vi "main_grid_forming_PQ.vi"() -> ()   [LabVIEW 2021]
uses:
  <vilib>/xnet/xnet.llb/XNET Frame CAN.ctl
  <vilib>/xnet/xnet.llb/XNET Frame Type CAN.ctl
  Helper functions/General Purpose/references.ctl
  Helper functions/General Purpose/measurements.ctl
  Helper functions/Time-sync/time_sync/TypeDef/Synch_shift--cluster.ctl
  <vilib>/Platform/TimedLoop/XDataNode/timing_clust.ctl
  <vilib>/Platform/TimedLoop/XDataNode/nitl_modes.ctl
  <vilib>/Platform/TimedLoop/XDataNode/wakeup.ctl
  Helper functions/communication/AFE_froming_Central.ctl
  Helper functions/communication/AFE_froming_Central_Info.ctl
  Helper functions/communication/AFE_froming_Central_Data.ctl
  <vilib>/xnet/xnet.llb/XNET Write (Frame CAN).vi
  <vilib>/xnet/xnet.llb/XNET Read (Frame CAN).vi
  <vilib>/Platform/TimedLoop/XDataNode/XDataNode.xnode
  <vilib>/Platform/TimedLoop/XDataNode/XDNodeRunTimeDep.lvlib
  <userlib>/_OpenG.lib/boolean/boolean.llb/openg_boolean__ogtk.lvlib
panel:
  in  "P2 bias":dbl
  in  "Calibration 2":T1={"IC1_Q_gain"=0.99511, "IC1_Q_bias"=-110.0, "IC2_Q_gain"=1.289, "IC2_Q_bias"=-368.5, "IC3_Q_gain"=1.003, "IC3_Q_bias"=-176.0, "IC2_P_gain"=1.2368, "IC2_P_bias"=1804.5, "IC3_P_gain"=0.9849, "IC3_P_bias"=1434.5}
  in  "Calibration":T1={"IC1_Q_gain"=0.997, "IC1_Q_bias"=-125.0, "IC2_Q_gain"=1.2829, "IC2_Q_bias"=-381.0, "IC3_Q_gain"=1.02, "IC3_Q_bias"=-252.4, "IC2_P_gain"=1.2775, "IC2_P_bias"=1561.0, "IC3_P_gain"=0.9939, "IC3_P_bias"=1271.0}
  in  "Q2 bias":dbl
  in  "delta V":dbl format="%#_13g"
  in  "delta f":dbl=0.005800000000000027 format="%#_13g"
  in  "biasQ4":dbl=200.0
  in  "biasV4":dbl
  in  "biasV1":dbl=0.6
  out "time_afe":timestamp
  out "start following 1 pre":bool
  out "Synch Monitor":string[][](table)
  in  "Loop Time":u32=125
  out "Error out":errorcluster
  in  "Timeout [ms]":i32=3000
  out "Offset from TR (ns)":dbl
  out "Status Out":T2
  out "CAN OUT":T3[](array[typedef]) {"payload" format="%x"; "timestamp" format="%<%.7X\n%x>T"; "type" items=["CAN Data"=0, "CAN Remote"=1, "CAN Bus Error"=2, "CAN 2.0 Data"=8, "CAN FD Data"=16, "CAN FD+BRS Data"=24, "J1939 Data"=192, "Delay"=224, "Log Trigger"=225, "Start Trigger"=226]; "identifier" format="%x"}
  in  "freq 1":dbl=50.0
  in  "Vabs 1":dbl=230.0
  in  "Varg 1":dbl
  in  "Start following 1":bool
  out "Forming 2":bool
  out "Forming 1":bool
  in  "Start forming 1":bool
  out "current time":timestamp
  in  "measurements":T5
  in  "references":T6
  in  "To ACT CH 4":bool
  in  "To ACT CH 3":bool
  in  "To ACT CH 2":bool
  out "Error 4":bool
  out "Fault 4":bool
  out "Error 3":bool
  out "Fault 3":bool
  out "Error 2":bool
  out "Fault 2":bool
  out "State code 4":i32
  out "State code 3":i32
  out "State code 2":i32
  out "State code 1":i32
  out "Error 1":bool
  out "Fault 1":bool
  in  "To ACT CH 1":bool
  in  "main stop":bool
  in  "Vdc4":dbl=750.0
  in  "Qac4":dbl
  in  "Pac3":dbl=750.0
  in  "Qac3":dbl
  in  "Pac2":dbl
  in  "Qac2":dbl
  in  "Emergency 4":bool
  in  "To IN OP  4":bool
  in  "SEND sp 4":bool
  in  "Clear 4":bool
  in  "Shutdwn 4":bool
  in  "Emergency 3":bool
  in  "To IN OP  3":bool
  in  "SEND sp 3":bool
  in  "Clear 3":bool
  in  "Shutdwn 3":bool
  in  "Emergency 2":bool
  in  "To IN OP  2":bool
  in  "SEND sp 2":bool
  in  "Clear 2":bool
  in  "Shutdwn 2":bool
  out "V slider 22":dbl(slide) caption="V-i" max=-10.0 scale=650.0..780.0 scale format="%#_4g"
  out "V slider 21":dbl(slide) caption="V-i" max=-10.0 scale=650.0..780.0 scale format="%#_4g"
  out "V slider 20":dbl(slide) caption="V-i" max=-10.0 scale=650.0..780.0 scale format="%#_4g"
  out "kW":dbl caption="Numeric" format="%#.3g"
  out "?VkVAr":dbl caption="Numeric" format="%.3g"
  out "kW":dbl caption="Numeric" format="%#.3g"
  out "?VkVAr":dbl caption="Numeric" format="%.3g"
  out "kW":dbl caption="Numeric" format="%#.3g"
  out "?VkVAr":dbl caption="Numeric" format="%.3g"
  out "OFF 4":bool
  out "ON 4":bool
  out "Ready 4":bool
  out "OFF 3":bool
  out "ON 3":bool
  out "Ready 3":bool
  out "OFF 2":bool
  out "ON 2":bool
  out "Ready 2":bool
  out "error out":errorcluster
  out "?VkVAr":dbl caption="Numeric" format="%.3g"
  out "kW":dbl caption="Numeric" format="%#.3g"
  out "V slider 19":dbl(slide) caption="V-i" max=-10.0 scale=650.0..780.0 scale format="%#_4g"
  in  "Vdc1":dbl=720.0
  out "OFF 1":bool
  out "ON 1":bool
  out "Ready 1":bool
  out "CAN IN":T3 {"payload" format="%x"; "timestamp" format="%<%.7X\n%x>T"; "type" items=["CAN Data"=0, "CAN Remote"=1, "CAN Bus Error"=2, "CAN 2.0 Data"=8, "CAN FD Data"=16, "CAN FD+BRS Data"=24, "J1939 Data"=192, "Delay"=224, "Log Trigger"=225, "Start Trigger"=226]; "identifier" format="%x"}
  in  "Emergency 1":bool
  in  "Qac1":dbl
  in  "conv":T7
  in  "CAN [ms]":i64=1
  out "CAN with Conv":bool
  out "Measurements":bool
  in  "Shutdwn 1":bool
  in  "Clear 1":bool
  in  "SEND sp 1":bool
  in  "To IN OP 1":bool
  out "logging":bool
  # "Resource agents: AFE 1-4"
  # "package identifiers:\n1xx VSC1 \n2xx VSC2\n3xx VSC3\n4xx VSC4\n\nx0x send from agent to resource\nx02 Power setpoints\nx06 Measurements\nx9 status\n          = [state; error; alarm; OFF; Ready; ON]\n\n \n\nx1x send from resource to agent\nx10 Power measurements\nx11 Measurements\nx12 status\n          = [state; error; alarm; full; precharge; neg; 0; 0]"
  # "B18"
  # "B 22\nB19"
  # "VSC 4"
  # "B17"
  # "B21"
  # "VSC 3"
  # "B16"
  # "B20"
  # "Start-up - Shut down"
  # "VSC 2"
  # "B15"
  # "B19"
  # "Start-up - Shut down"
  # "VSC 1"
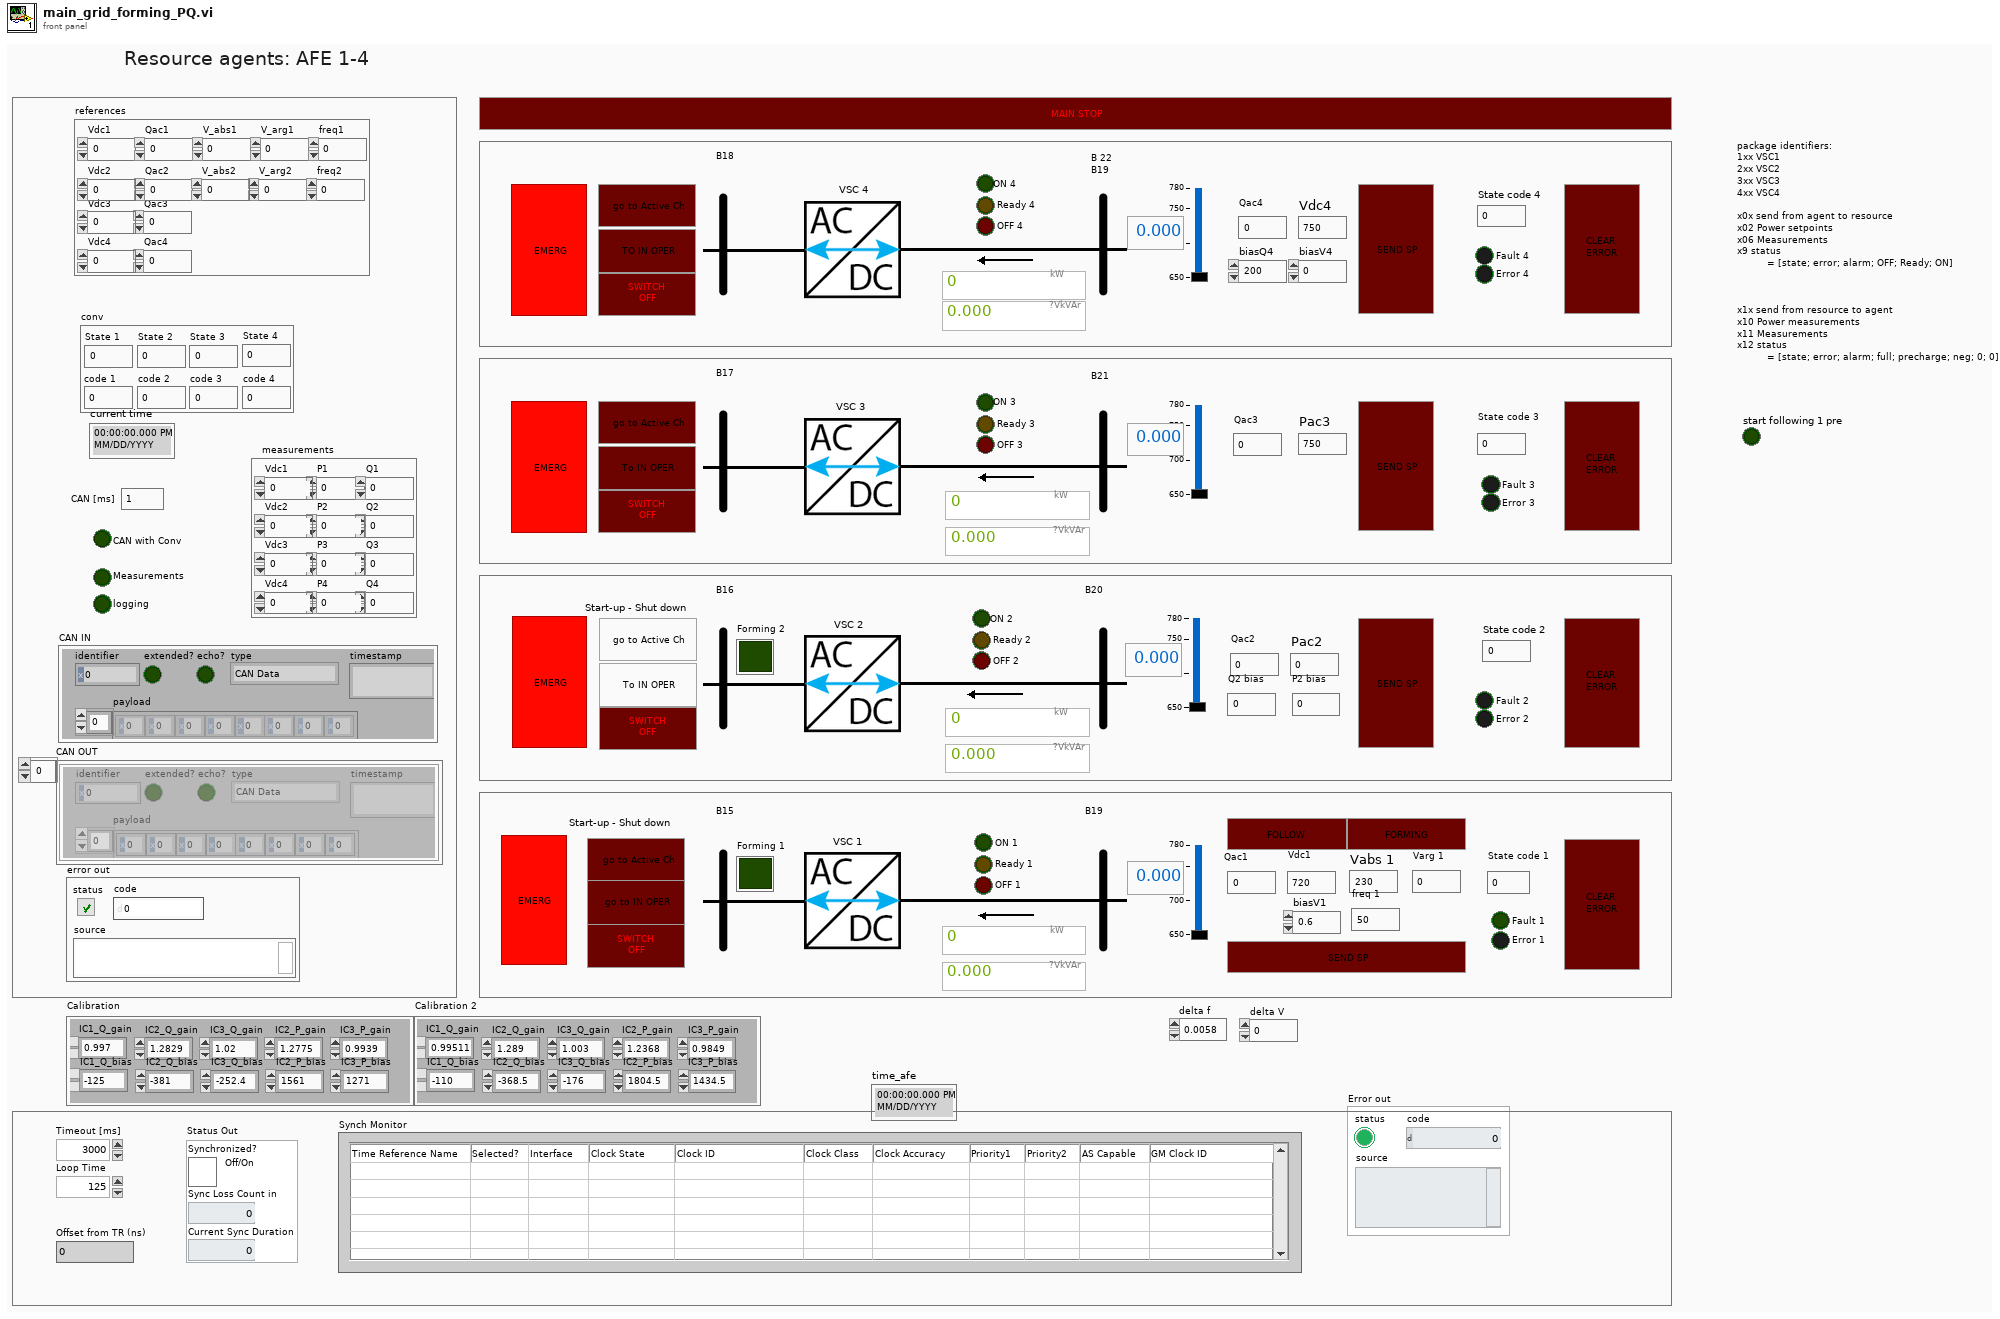
[diagram p1: front panel]
types:
  T1 = cluster{"IC1_Q_gain":dbl, "IC1_Q_bias":dbl, "IC2_Q_gain":dbl, "IC2_Q_bias":dbl, "IC3_Q_gain":dbl, "IC3_Q_bias":dbl, "IC2_P_gain":dbl, "IC2_P_bias":dbl, "IC3_P_gain":dbl, "IC3_P_bias":dbl}
  T2 = typedef "Synch_shift--cluster.ctl" = cluster{"Synchronized?":bool, "Sync Loss Count in":u32, "Current Sync Duration":u32}
  T3 = typedef "XNET Frame CAN.ctl" = cluster{"timestamp":timestamp, "payload":u8[], "identifier":u32, "type":T4, "extended?":bool, "echo?":bool}
  T4 = typedef "XNET Frame Type CAN.ctl" = u8
  T5 = typedef "measurements.ctl" = cluster{"Vdc1":dbl, "P1":dbl, "Vdc2":dbl, "P2":dbl, "Q2":dbl, "Vdc3":dbl, "P3":dbl, "Q3":dbl, "Vdc4":dbl, "P4":dbl, "Q4":dbl, "Q1":dbl}
  T6 = typedef "references.ctl" = cluster{"Vdc1":dbl, "Vdc2":dbl, "Qac2":dbl, "Vdc3":dbl, "Qac3":dbl, "Vdc4":dbl, "Qac4":dbl, "Qac1":dbl, "V_arg2":dbl, "V_abs2":dbl, "V_abs1":dbl, "V_arg1":dbl, "freq1":dbl, "freq2":dbl}
  T7 = cluster{"State 1":dbl, "code 1":dbl, "code 2":dbl, "code 3":dbl, "code 4":dbl, "State 2":dbl, "State 3":dbl, "State 4":dbl}
  T8 = cluster{"Frame In":refnum<k21>, "Frame Out":refnum<k21>}
  T9 = typedef "XDNodeRunTimeDep.lvlib/timing_clust.ctl" = cluster{"Expected End [f-1]":u64, "Actual End [f-1]":u64, "Finished Late? [f-1]":bool, "Expected End [i-1]":u64, "Actual End [i-1]":u64, "Finished Late? [i-1]":bool, "Expected Start [i]":u64, "Actual Start [i]":u64, "Expected Start [f]":u64, "Actual Start [f]":u64, "Source Name":string, "Structure Name":string, "Period":i64, "Deadline":i64, "Offset":i64, "Start":i64, "Priority":i32, "Timeout":i32, "Mode":T10, "Wakeup Reason":T11, "Error":errorcluster, "Source Type":string, "Secondary Source Type":string, "Global End Time":u64, "Global Start Time":u64, "Frame Duration":u64, "Iteration Duration":u64, "Assigned CPU":i32, "I/O Scan Engine Mode":u32}
  T10 = typedef "XDNodeRunTimeDep.lvlib/nitl_modes.ctl" = enum32{"No Change", "Process missed periods, maintain original phase", "Discard missed periods, maintain original phase", "Process missed periods, ignore original phase", "Discard missed periods, ignore original phase"}
  T11 = typedef "XDNodeRunTimeDep.lvlib/wakeup.ctl" = enum32{"Normal", "Aborted", "Asynchronous wakeup", "Timing source error", "Timed loop error", "Timeout"}
  T12 = typedef "AFE_froming_Central.ctl" = cluster{"Info":T13, "Data":T14}
  T13 = typedef "AFE_froming_Central_Info.ctl" = cluster{"Resource":string, "Problem":bool, "Timestamp":dbl}
  T14 = typedef "AFE_froming_Central_Data.ctl" = cluster{"Start forming 1":bool, "Forming/Following":bool[], "Start forming 2":bool, "measurements":cluster{"Vdc1":dbl, "P1":dbl, "Vdc2":dbl, "P2":dbl, "Q2":dbl, "Vdc3":dbl, "P3":dbl, "Q3":dbl, "Vdc4":dbl, "P4":dbl, "Q4":dbl, "Q1":dbl}, "Status":bool[], "references":T6, "Start following 1":bool, "Start following 2":bool}
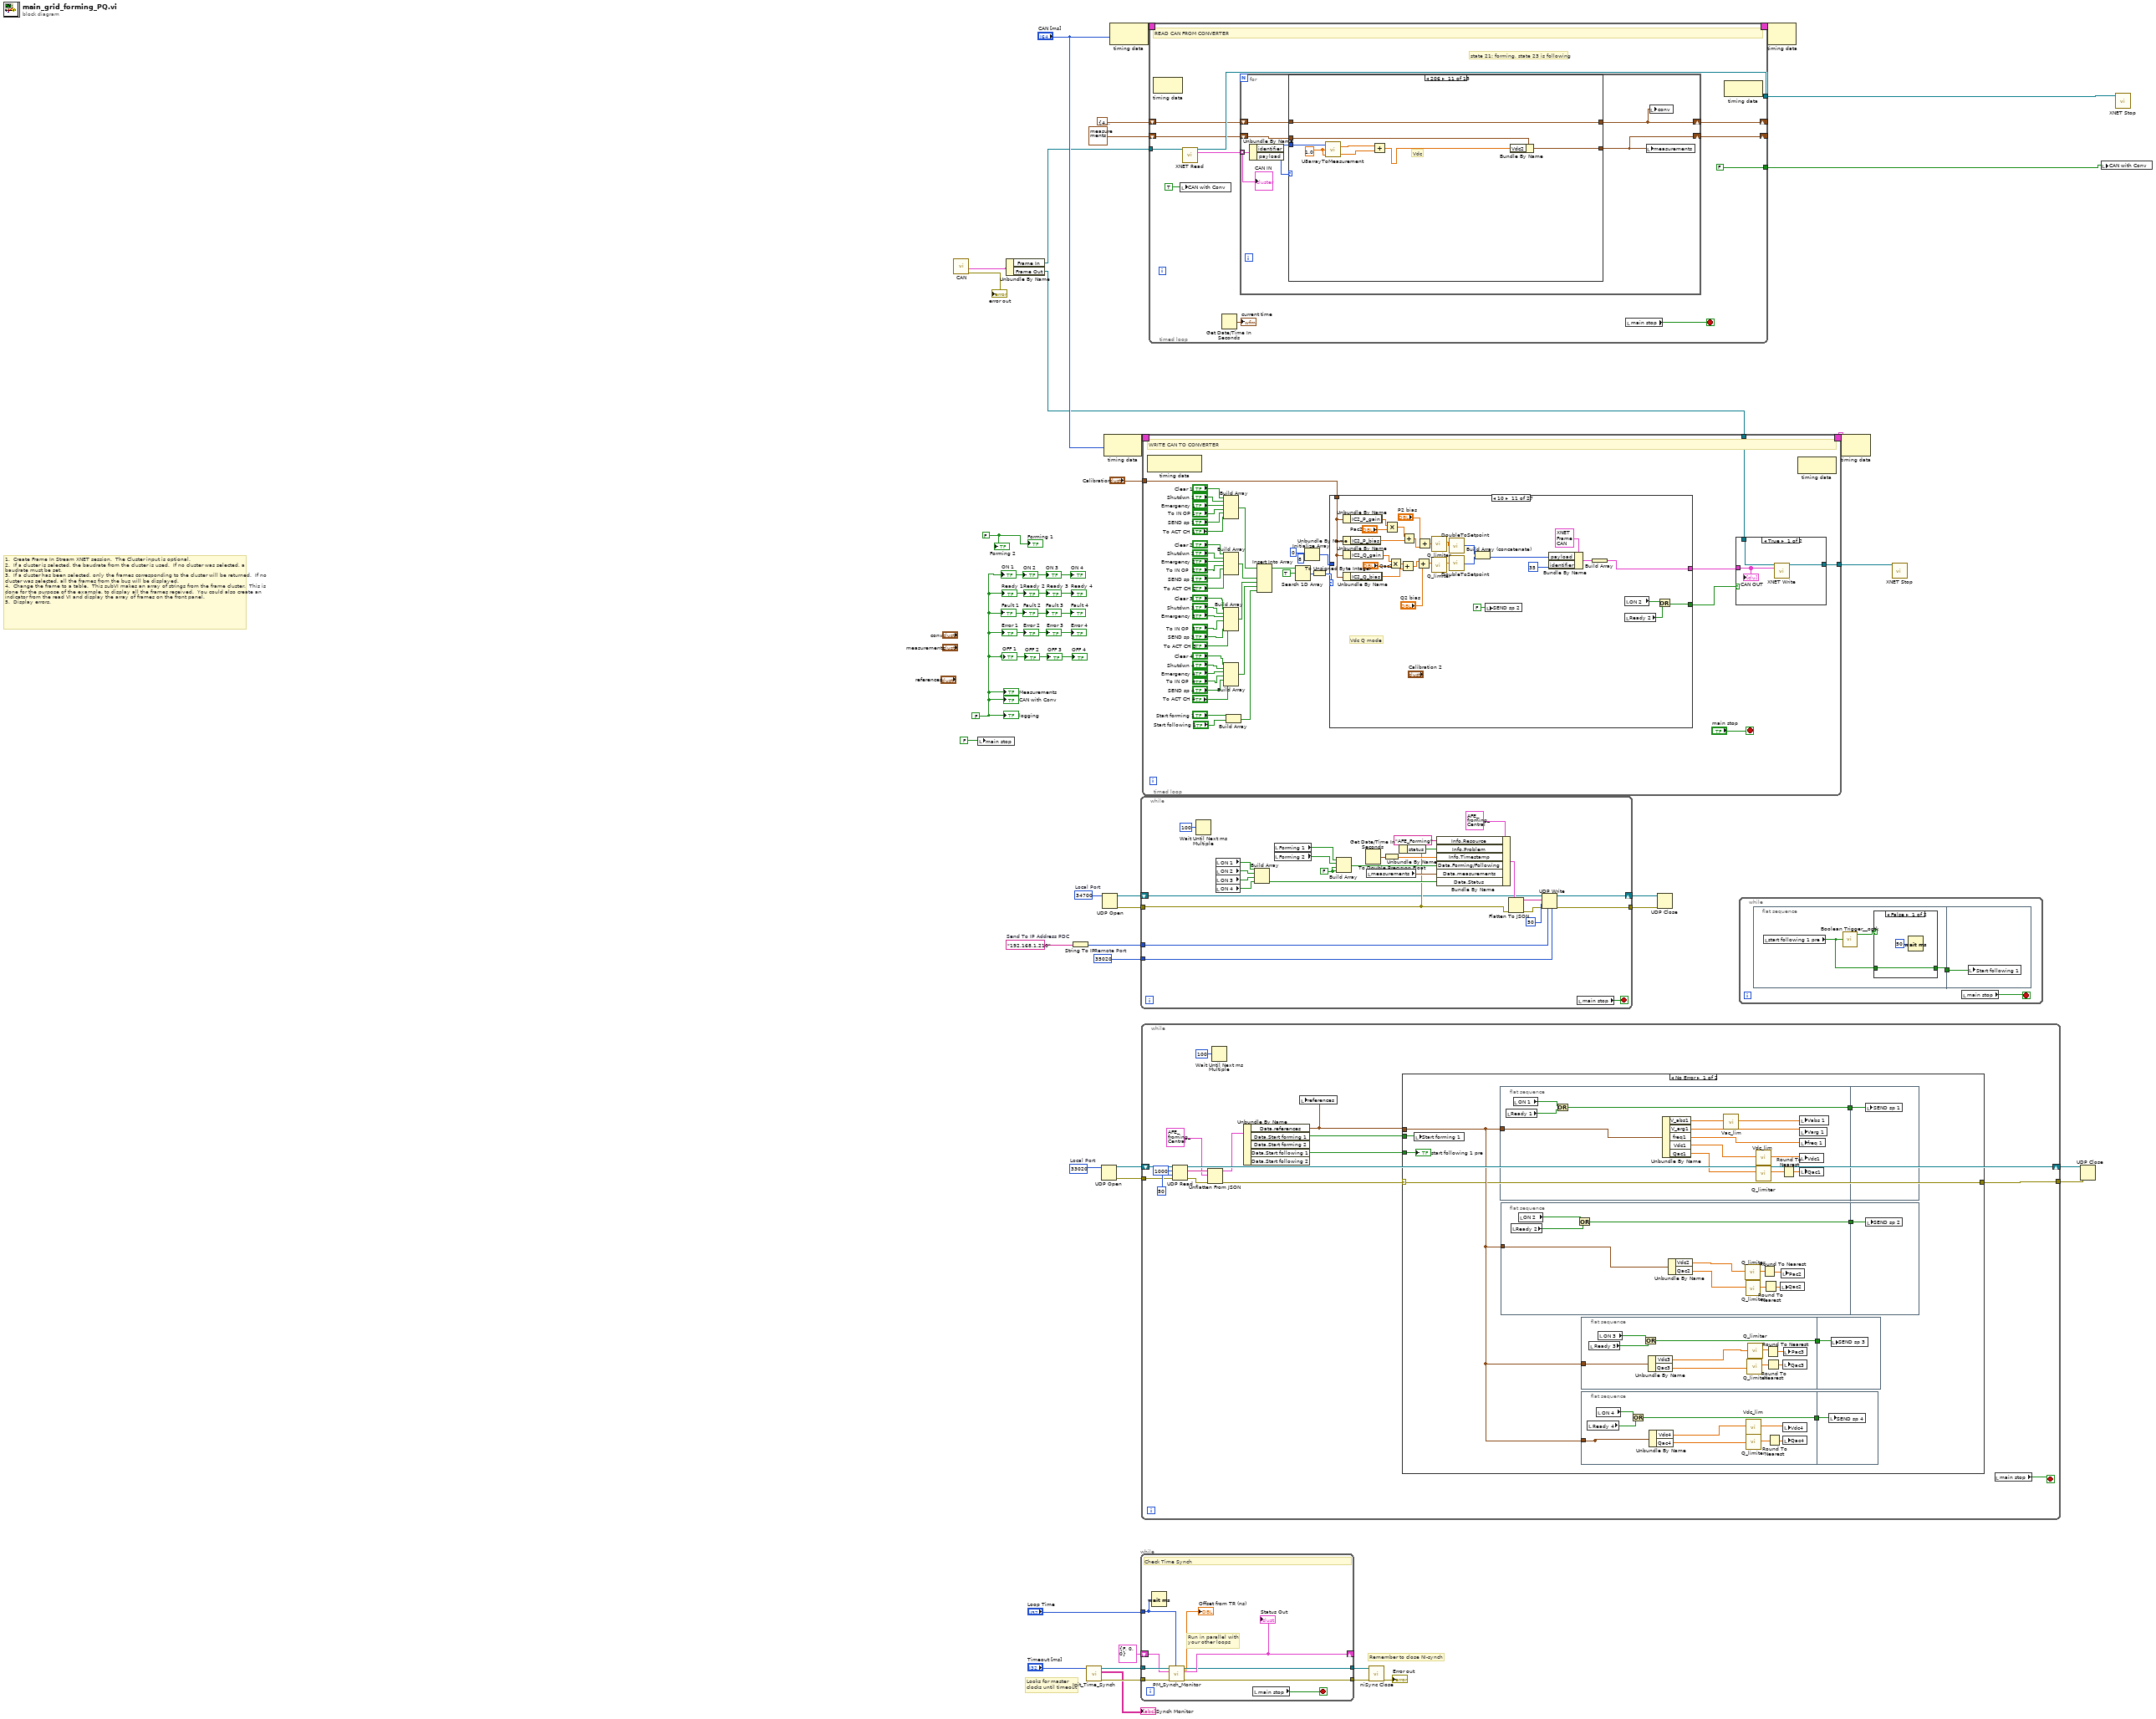
[diagram p0: block diagram]
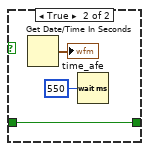
[diagram p2: hidden frame]
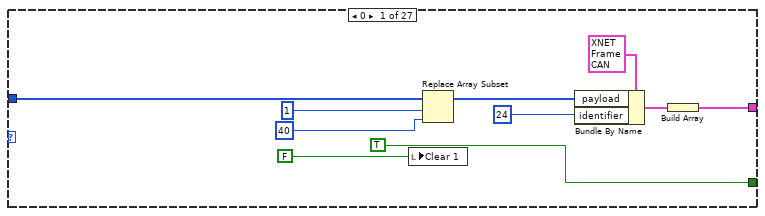
[diagram p5: hidden frame]
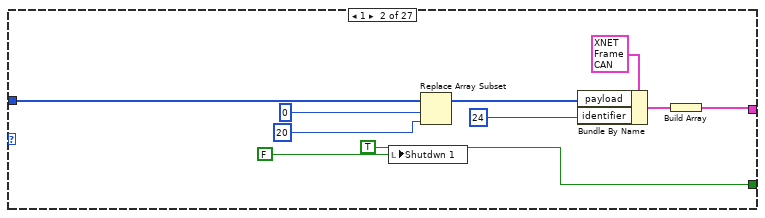
[diagram p6: hidden frame]
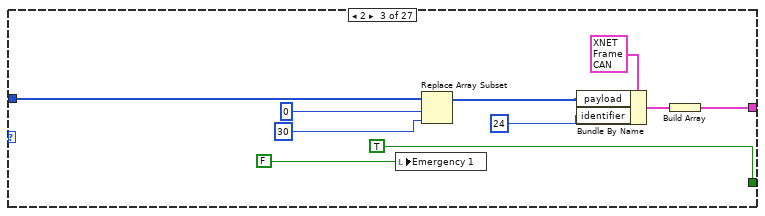
[diagram p7: hidden frame]
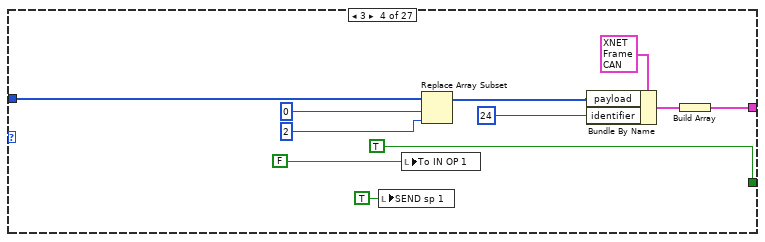
[diagram p8: hidden frame]
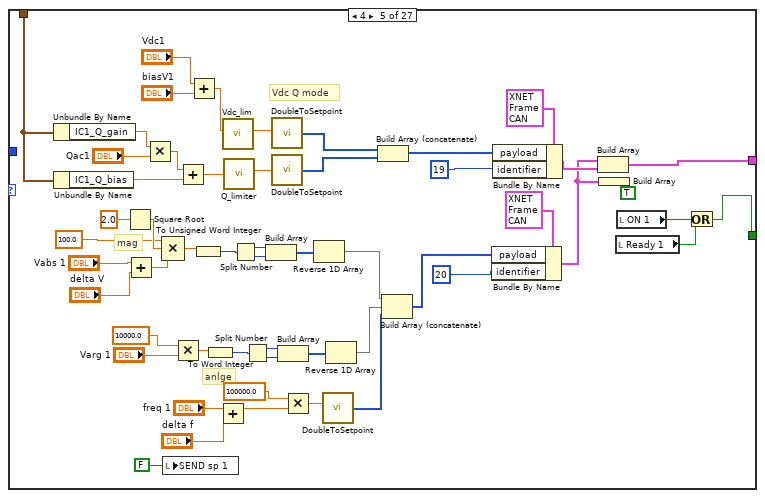
[diagram p9: hidden frame]
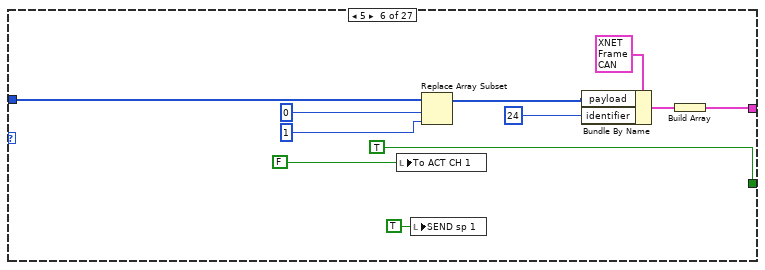
[diagram p10: hidden frame]
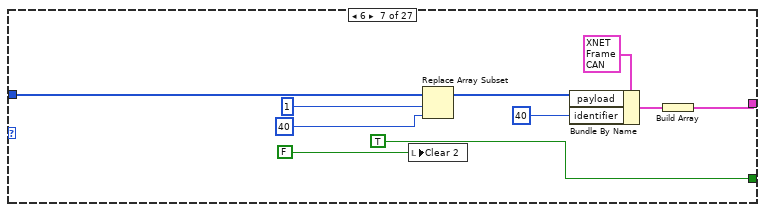
[diagram p11: hidden frame]
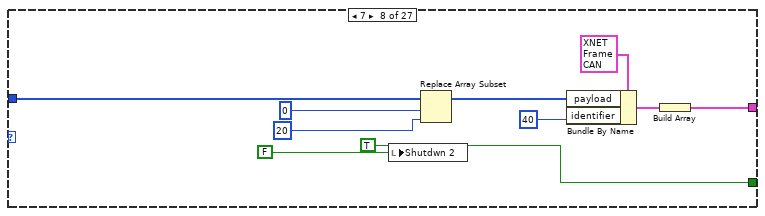
[diagram p12: hidden frame]
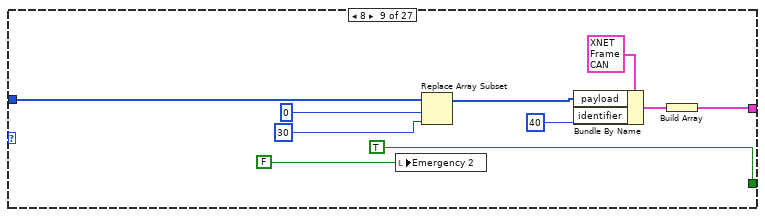
[diagram p13: hidden frame]
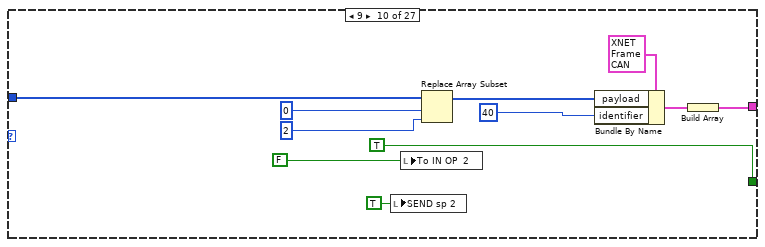
[diagram p14: hidden frame]
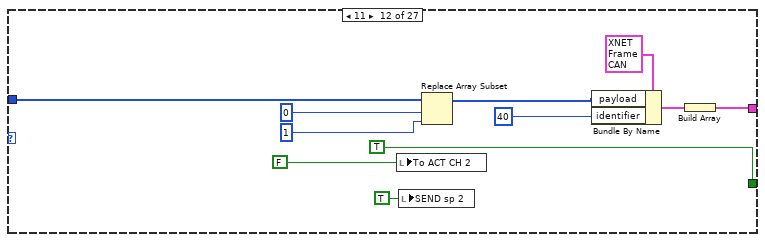
[diagram p15: hidden frame]
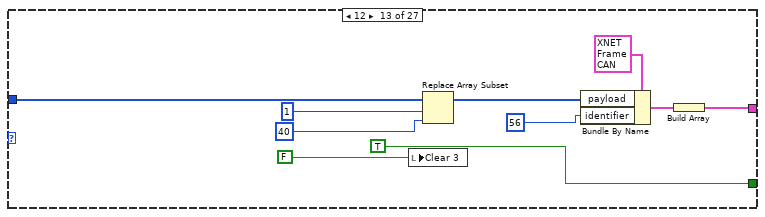
[diagram p16: hidden frame]
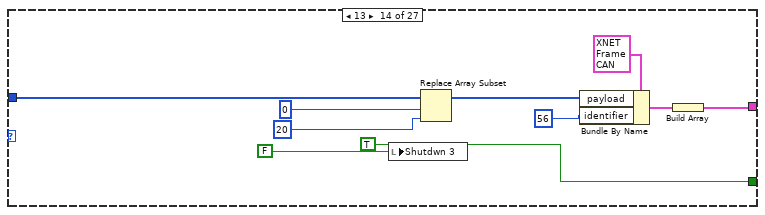
[diagram p17: hidden frame]
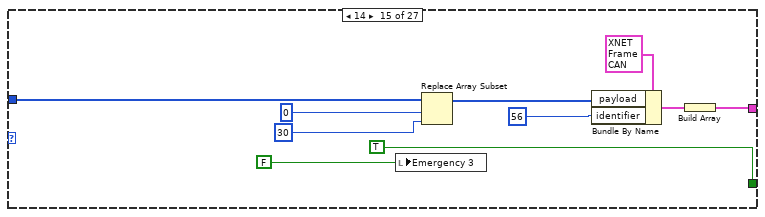
[diagram p18: hidden frame]
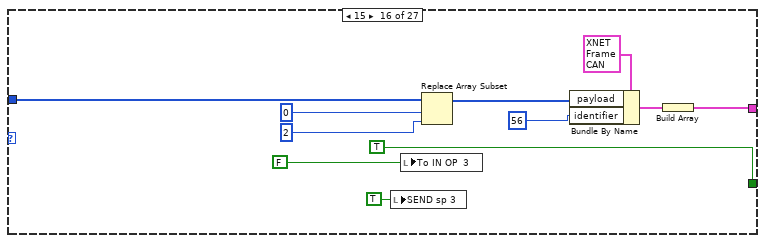
[diagram p19: hidden frame]
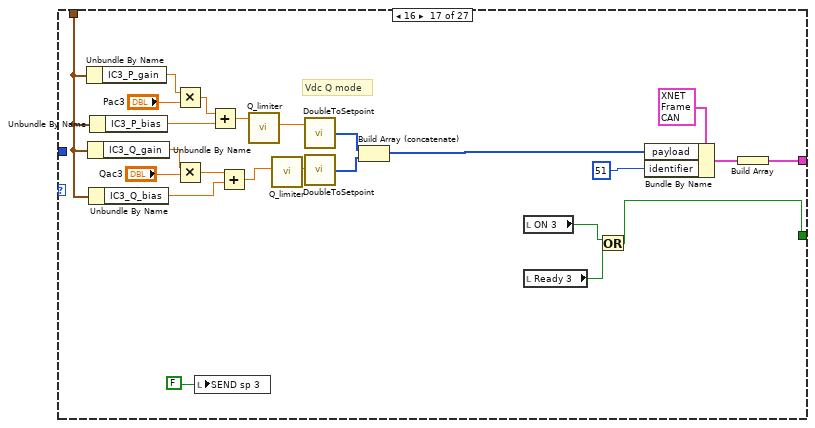
[diagram p20: hidden frame]
diagram:
  w12 = u16 33020  # Local Port
  w23 = FALSE ("Forming")
  w6 = u16 35020  # Remote Port
  w24 = "192.168.1.210"  # Send To IP Address PDC
  w25 = u16 34700  # Local Port
  w26 = FALSE
  # "Remember to close NI-synch"
  # "Looks for master \nclocks until timeout"
  # "1.  Create Frame In Stream XNET session.  The Cluster input is optional.  \n2.  If a cluster is selected, the baudrate from the cluster is used.  If no cluster was selected, a baudrate must be set.\n3.  If a cluster has been selected, only the frames corresponding to the cluster will be returned.  If no cluster was selected, all the frames from the bus will be displayed.\n4.  Change the frame to a table.  This subVI makes an array of strings from the frame cluster.  This is done for the purpose of the example, to display all the frames received.  You could also create an indicator from the read VI and display the array of frames on the front panel. \n5.  Display errors."
  n1 = call "CAN.vi"() -> ("error out"=→"error out":errorcluster, "CAN"=w28:T8)  [unwired: 10 in]
  n2 = local write "main stop"(FALSE ("main stop")) -> ()
  n3 = Unbundle By Name(w28) -> ("Frame In"=w33:refnum<k21>, "Frame Out"=w36:refnum<k21>)
  n4 = String To IP(1:w24) -> (0:w7:u32)
  n5 = call "Init_Time_Synch.vi"("Timeout [ms]"="Timeout [ms]") -> ("Error out"=w20:errorcluster, "Synch Monitor"=→"Synch Monitor":string[][], "Synch Out"=w18:refnum<k15>)  [unwired: 7 in, 1 out]
  n6 = UDP Open(11:w12) -> (port=w11:refnum<k16>, 0:w10:errorcluster)  [unwired: 4 in, 1 out]
  n7 = UDP Open(11:w25) -> (port=w5:refnum<k16>, 0:w4:errorcluster)  [unwired: 4 in, 1 out]
  n8 = node-c288("CAN [ms]") -> (w30:T9)
  n9 = node-c288("CAN [ms]") -> (w35:T9)
  n10 = while {
    tunnel: [w48] -> w8
    tunnel: w7 -> [w46]
    tunnel: w6 -> [w47]
    tunnel: w4 -> [w45]
    shift-right: [w43] -> w3
    shift-left: w5 -> [w44]
    stop <- w42 stop-if-true
    w65 = FALSE ("ON 1")
    n11 = Wait Until Next ms Multiple(millisecond multiple=u32 100) -> ()  [unwired: 1 out]
    n12 = local read "ON 1"() -> (w58:bool)
    n13 = local read "ON 2"() -> (w57:bool)
    n14 = local read "ON 3"() -> (w59:bool)
    n15 = local read "ON 4"() -> (w60:bool)
    n16 = Build Array(w58, w57, w59, w60) -> (w61:bool[])
    n17 = local read "Forming 1"() -> (w64:bool)
    n18 = local read "Forming 2"() -> (w63:bool)
    n19 = Build Array(w64, w63, w65, w65) -> (w62:bool[])
    n20 = Get Date/Time In Seconds() -> (seconds since 1Jan1904=w53:timestamp)
    n21 = local read "measurements"() -> (w56:T5)
    n22 = To Double Precision Float(number=w53) -> (double precision float=w54:dbl)
    n23 = Unbundle By Name(w45) -> ("status"=w66:bool)
    n24 = Bundle By Name(cluster=T12 {"Info"={"Resource"="AFE_Forming", "Problem"=FALSE, "Timestamp"=0.0}, "Data"={"Start forming 1"=FALSE, "Forming/Following"=[], "Start forming 2"=FALSE, "measurements"={"Vdc1"=0.0, "P1"=0.0, "Vdc2"=0.0, "P2"=0.0, "Q2"=0.0, "Vdc3"=0.0, "P3"=0.0, "Q3"=0.0, "Vdc4"=0.0, "P4"=0.0, "Q4"=0.0, "Q1"=0.0}, "Status"=[], "references"={"Vdc1"=0.0, "Vdc2"=0.0, "Qac2"=0.0, "Vdc3"=0.0, "Qac3"=0.0, "Vdc4"=0.0, "Qac4"=0.0, "Qac1"=0.0, "V_arg2"=0.0, "V_abs2"=0.0, "V_abs1"=0.0, "V_arg1"=0.0, "freq1"=0.0, "freq2"=0.0}, "Start following 1"=FALSE, "Start following 2"=FALSE}} ("Cluster"), "Info.Resource"="AFE_Forming", "Info.Problem"=w66, "Info.Timestamp"=w54, "Data.Forming/Following"=w62, "Data.measurements"=w56, "Data.Status"=w61) -> (w67:T12)
    n25 = Flatten To JSON(anything=w67, error in (no error)=w45) -> (JSON string=w51:string, 11:w52:errorcluster)  [unwired: 1 in]
    n26 = UDP Write(address=w46, port or service name=w47, connection ID=w44, data in=w51, 8:w52, 9:50 ("timeout ms (25000)")) -> (error out=w48:errorcluster, 3:w43:refnum<k16>)
    n27 = local read "main stop"() -> (w42:bool)
  }
  n28 = while {
    tunnel: w20 -> [w72]
    tunnel: [w73] -> w15
    shift-right: [w74] -> _
    shift-left: T2 {"Synchronized?"=FALSE, "Sync Loss Count in"=0, "Current Sync Duration"=0} ("Status In") -> [w75]
    tunnel: w18 -> [w76]
    tunnel: "Loop Time" -> [w69]
    tunnel: [w71] -> w16
    stop <- w68 stop-if-true
    # "Run in parallel with \nyour other loops"
    # "Check Time Synch"
    n29 = Wait (ms)(milliseconds to wait=w69) -> ()  [unwired: 1 out]
    n30 = call "PM_Synch_Monitor.vi"("Polling Interval"=w69, "error in"=w72, "Status In"=w75, "Synch In"=w76) -> ("error out"=w73:errorcluster, "Status Out"=w74:T2, "Reference out"=w71:refnum<k15>, "Offset from TR (ns)"=→"Offset from TR (ns)":dbl)  [unwired: 3 in, 1 out]
    "Status Out" <- w74
    n31 = local read "main stop"() -> (w68:bool)
  }
  n32 = while {
    tunnel: w10 -> [w81]
    shift-right: [w89] -> w9
    shift-left: w11 -> [w82]
    tunnel: [w78] -> w2
    stop <- w92 stop-if-true
    n33 = UDP Read(connection ID=w82, max size (548)=1000, timeout ms (25000)=50, 8:w81) -> (data out=w88:string, error out=w86:errorcluster, 3:w89:refnum<k16>)  [unwired: 2 out]
    n34 = Unflatten From JSON(JSON string=w88, type and defaults=T12 {"Info"={"Resource"="AFE_Forming", "Problem"=FALSE, "Timestamp"=0.0}, "Data"={"Start forming 1"=FALSE, "Forming/Following"=[], "Start forming 2"=FALSE, "measurements"={"Vdc1"=0.0, "P1"=0.0, "Vdc2"=0.0, "P2"=0.0, "Q2"=0.0, "Vdc3"=0.0, "P3"=0.0, "Q3"=0.0, "Vdc4"=0.0, "P4"=0.0, "Q4"=0.0, "Q1"=0.0}, "Status"=[], "references"={"Vdc1"=0.0, "Vdc2"=0.0, "Qac2"=0.0, "Vdc3"=0.0, "Qac3"=0.0, "Vdc4"=0.0, "Qac4"=0.0, "Qac1"=0.0, "V_arg2"=0.0, "V_abs2"=0.0, "V_abs1"=0.0, "V_arg1"=0.0, "freq1"=0.0, "freq2"=0.0}, "Start following 1"=FALSE, "Start following 2"=FALSE}} ("Cluster"), error in (no error)=w86) -> (value=w85:T12, error out=w90:errorcluster)  [unwired: 4 in]
    n35 = Wait Until Next ms Multiple(millisecond multiple=u32 100) -> ()  [unwired: 1 out]
    n36 = Unbundle By Name(w85) -> ("Data.references"=w91:T6, "Data.Start forming 1"=w79:bool, "Data.Start following 1"=w80:bool)  [unwired: 2 out]
    n37 = local write "references"(w91) -> ()
    n38 = case shown="No Error" w90 {
      selector: w90 -> [w93 w147]
      tunnel: w91 -> [w100 _]
      tunnel: w80 -> [w95 _]
      tunnel: w79 -> [w94 _]
      tunnel: [w93 w147] -> w78
      frame No Error {
        n39 = local write "Start forming 1"(w94) -> ()
        n40 = flat-sequence {
          tunnel: w100 -> [w145]
          tunnel: [w135] -> w98
          tunnel: w98 -> [w146]
          frame #0 {
            n41 = local read "Ready 1"() -> (w137:bool)
            n42 = local read "ON 1"() -> (w136:bool)
            n43 = Or(x=w136, y=w137) -> (x .or. y?=w135:bool)
            n44 = Unbundle By Name(w145) -> ("V_abs1"=w143:dbl, "V_arg1"=w144:dbl, "freq1"=w141:dbl, "Vdc1"=w133:dbl, "Qac1"=w138:dbl)
            n45 = call "Vac_lim.vi"("IN Vdc"=w143) -> ("OUT Vdc"=w142:dbl)  [unwired: 10 in]
            n46 = call "Vdc_lim.vi"("IN Vdc"=w133) -> ("OUT Vdc"=w140:dbl)  [unwired: 10 in]
            n47 = call "Q_limiter.vi"("IN Q"=w138) -> ("OUT Q"=w139:dbl)  [unwired: 10 in]
            n48 = Round To Nearest(number=w139) -> (nearest integer value=w134:dbl)
            n49 = local write "Vabs 1"(w142) -> ()
            n50 = local write "Varg 1"(w144) -> ()
            n51 = local write "freq 1"(w141) -> ()
            n52 = local write "Vdc1"(w140) -> ()
            n53 = local write "Qac1"(w134) -> ()
          }
          frame #1 {
            n54 = local write "SEND sp 1"(w146) -> ()
          }
        }
        n55 = flat-sequence {
          tunnel: w100 -> [w131]
          tunnel: [w126] -> w99
          tunnel: w99 -> [w132]
          frame #0 {
            n56 = local read "Ready 2"() -> (w128:bool)
            n57 = local read "ON 2"() -> (w127:bool)
            n58 = Or(x=w127, y=w128) -> (x .or. y?=w126:bool)
            n59 = Unbundle By Name(w131) -> ("Vdc2"=w122:dbl, "Qac2"=w129:dbl)
            n60 = call "Q_limiter.vi"("IN Q"=w122) -> ("OUT Q"=w123:dbl)  [unwired: 10 in]
            n61 = call "Q_limiter.vi"("IN Q"=w129) -> ("OUT Q"=w130:dbl)  [unwired: 10 in]
            n62 = Round To Nearest(number=w123) -> (nearest integer value=w124:dbl)
            n63 = Round To Nearest(number=w130) -> (nearest integer value=w125:dbl)
            n64 = local write "Qac2"(w125) -> ()
            n65 = local write "Pac2"(w124) -> ()
          }
          frame #1 {
            n66 = local write "SEND sp 2"(w132) -> ()
          }
        }
        n67 = flat-sequence {
          tunnel: w100 -> [w120]
          tunnel: [w117] -> w97
          tunnel: w97 -> [w121]
          frame #0 {
            n68 = local read "Ready 3"() -> (w118:bool)
            n69 = local read "ON 3"() -> (w116:bool)
            n70 = Or(x=w116, y=w118) -> (x .or. y?=w117:bool)
            n71 = Unbundle By Name(w120) -> ("Vdc3"=w113:dbl, "Qac3"=w119:dbl)
            n72 = call "Q_limiter.vi"("IN Q"=w119) -> ("OUT Q"=w115:dbl)  [unwired: 10 in]
            n73 = call "Q_limiter.vi"("IN Q"=w113) -> ("OUT Q"=w112:dbl)  [unwired: 10 in]
            n74 = Round To Nearest(number=w112) -> (nearest integer value=w111:dbl)
            n75 = Round To Nearest(number=w115) -> (nearest integer value=w114:dbl)
            n76 = local write "Qac3"(w114) -> ()
            n77 = local write "Pac3"(w111) -> ()
          }
          frame #1 {
            n78 = local write "SEND sp 3"(w121) -> ()
          }
        }
        n79 = flat-sequence {
          tunnel: [w109] -> _
          tunnel: w100 -> [w109]
          tunnel: [w103] -> w96
          tunnel: w96 -> [w110]
          frame #0 {
            n80 = local read "Ready 4"() -> (w105:bool)
            n81 = local read "ON 4"() -> (w104:bool)
            n82 = Or(x=w104, y=w105) -> (x .or. y?=w103:bool)
            n83 = Unbundle By Name(w109) -> ("Vdc4"=w101:dbl, "Qac4"=w106:dbl)
            n84 = call "Vdc_lim.vi"("IN Vdc"=w101) -> ("OUT Vdc"=w108:dbl)  [unwired: 10 in]
            n85 = call "Q_limiter.vi"("IN Q"=w106) -> ("OUT Q"=w107:dbl)  [unwired: 10 in]
            n86 = Round To Nearest(number=w107) -> (nearest integer value=w102:dbl)
            n87 = local write "Vdc4"(w108) -> ()
            n88 = local write "Qac4"(w102) -> ()
          }
          frame #1 {
            n89 = local write "SEND sp 4"(w110) -> ()
          }
        }
        "start following 1 pre" <- w95
      }
      frame Error {
      }
    }
    n90 = local read "main stop"() -> (w92:bool)
  }
  n91 = timed-loop {
    tunnel: w36 -> [w188]
    tunnel: [w187] -> w39
    timing: w30 -> [_]
    timing-out: [_] -> w29
    tunnel: "Calibration" -> [w148]
    stop <- "main stop" stop-if-true
    # "WRITE CAN TO CONVERTER"
    n92 = node-c288() -> ()  [unwired: 1 in, 1 out]
    n93 = Build Array("Clear 1", "Shutdwn 1", "Emergency 1", "To IN OP 1", "SEND sp 1", "To ACT CH 1") -> (w163:bool[])
    n94 = Build Array("Clear 2", "Shutdwn 2", "Emergency 2", "To IN OP  2", "SEND sp 2", "To ACT CH 2") -> (w162:bool[])
    n95 = Build Array("Clear 3", "Shutdwn 3", "Emergency 3", "To IN OP  3", "SEND sp 3", "To ACT CH 3") -> (w161:bool[])
    n96 = Build Array("Clear 4", "Shutdwn 4", "Emergency 4", "To IN OP  4", "SEND sp 4", "To ACT CH 4") -> (w160:bool[])
    n97 = Build Array("Start forming 1", "Start following 1") -> (w154:bool[])
    n98 = Insert Into Array(array=w163, new element #1=w162, new element #2=w161, new element #3=w160, new element #4=w154) -> (w159:bool[])  [unwired: 1 in]
    n99 = Search 1D Array(1D array=w159, element=TRUE) -> (index of element=w181:i32)  [unwired: 1 in]
    n100 = Initialize Array(u8 0, 8 ("dimension size")) -> (w189:u8[])
    n101 = To Unsigned Byte Integer(number=w181) -> (unsigned 8bit integer=w185:u8)
    n102 = case shown="10" w185 {
      tunnel: w189 -> [w205 w215 w225 w236 _ w299 w309 w319 w329 w340 _ w379 w389 w399 w409 w420 _ w455 w465 w475 w485 w496 _ w526 w538 w552 w554]
      tunnel: [TRUE TRUE TRUE TRUE w288 TRUE TRUE TRUE TRUE TRUE w367 TRUE TRUE TRUE TRUE TRUE w443 TRUE TRUE TRUE TRUE TRUE w513 TRUE w529 TRUE FALSE] -> w153
      tunnel: [w197 w209 w217 w228 w255 w292 w301 w312 w321 w332 w362 w372 w381 w391 w401 w412 w437 w446 w459 w469 w479 w488 w508 w517 w531 w544 w556] -> w152
      tunnel: w148 -> [_ _ _ _ w238 _ _ _ _ _ w345 _ _ _ _ _ w422 _ _ _ _ _ _ _ _ _ _]
      frame 0 {
        n103 = local write "Clear 1"(FALSE ("Clear")) -> ()
        n104 = Replace Array Subset(array=w205, new element=u8 40 ("new element/subarray"), index=1) -> (w199:u8[])
        n105 = Bundle By Name(cluster=T3 {"timestamp"=timestamp(0 s since 1904-01-01), "payload"=[], "identifier"=0, "type"=0, "extended?"=FALSE, "echo?"=FALSE} ("CAN frame 3"), "payload"=w199, "identifier"=u32 24) -> (w200:T3)
        n106 = Build Array(w200) -> (w197:T3[])
      }
      frame 1 {
        n107 = local write "Shutdwn 1"(FALSE ("Shutdwn")) -> ()
        n108 = Replace Array Subset(array=w215, new element=u8 20 ("new element/subarray"), index=0) -> (w208:u8[])
        n109 = Bundle By Name(cluster=T3 {"timestamp"=timestamp(0 s since 1904-01-01), "payload"=[], "identifier"=0, "type"=0, "extended?"=FALSE, "echo?"=FALSE} ("CAN frame 3"), "payload"=w208, "identifier"=u32 24) -> (w210:T3)
        n110 = Build Array(w210) -> (w209:T3[])
      }
      frame 2 {
        n111 = local write "Emergency 1"(FALSE ("Idc cmd")) -> ()
        n112 = Replace Array Subset(array=w225, new element=u8 30 ("new element/subarray"), index=0) -> (w219:u8[])
        n113 = Bundle By Name(cluster=T3 {"timestamp"=timestamp(0 s since 1904-01-01), "payload"=[], "identifier"=0, "type"=0, "extended?"=FALSE, "echo?"=FALSE} ("CAN frame 3"), "payload"=w219, "identifier"=u32 24) -> (w220:T3)
        n114 = Build Array(w220) -> (w217:T3[])
      }
      frame 3 {
        n115 = local write "SEND sp 1"(TRUE ("SEND sp 1")) -> ()
        n116 = local write "To IN OP 1"(FALSE ("Idc cmd")) -> ()
        n117 = Replace Array Subset(array=w236, new element=u8 2 ("new element/subarray"), index=0) -> (w229:u8[])
        n118 = Bundle By Name(cluster=T3 {"timestamp"=timestamp(0 s since 1904-01-01), "payload"=[], "identifier"=0, "type"=0, "extended?"=FALSE, "echo?"=FALSE} ("CAN frame 3"), "payload"=w229, "identifier"=u32 24) -> (w231:T3)
        n119 = Build Array(w231) -> (w228:T3[])
      }
      frame 4 {
        (unwired) TRUE
        # "anlge"
        # "mag"
        # "Vdc Q mode"
        n120 = Unbundle By Name(w238) -> ("IC1_Q_gain"=w239:dbl)
        n121 = Unbundle By Name(w238) -> ("IC1_Q_bias"=w240:dbl)
        n122 = Square Root(x=2.0) -> (sqrt(x)=w254:dbl)
        n123 = Add(x="Vabs 1", y="delta V") -> (x+y=w246:dbl)
        n124 = Multiply(x=w239, y="Qac1") -> (x*y=w243:dbl)
        n125 = Compound Arithmetic op=MULTIPLY(100.0 ("value"), w254, w246) -> (w252:dbl)
        n126 = local write "SEND sp 1"(FALSE ("SEND sp")) -> ()
        n127 = Multiply(x=10000.0, y="Varg 1") -> (x*y=w264:dbl)
        n128 = Add(x=w243, y=w240) -> (x+y=w242:dbl)
        n129 = Add(x="Vdc1", y="biasV1") -> (x+y=w250:dbl)
        n130 = To Unsigned Word Integer(number=w252) -> (unsigned 16bit integer=w269:u16)
        n131 = To Word Integer(number=w264) -> (16bit integer=w265:i16)
        n132 = Add(x="freq 1", y="delta f") -> (x+y=w248:dbl)
        n133 = call "Vdc_lim.vi"("IN Vdc"=w250) -> ("OUT Vdc"=w280:dbl)  [unwired: 10 in]
        n134 = call "Q_limiter.vi"("IN Q"=w242) -> ("OUT Q"=w279:dbl)  [unwired: 10 in]
        n135 = Split Number(x=w269) -> (hi(x)=w270:u8, lo(x)=w271:u8)
        n136 = Split Number(x=w265) -> (hi(x)=w266:u8, lo(x)=w267:u8)
        n137 = Build Array(w270, w271) -> (w272:u8[])
        n138 = call "DoubleToSetpoint.vi"("Double"=w280) -> ("SP"=w282:u8[])
        n139 = call "DoubleToSetpoint.vi"("Double"=w279) -> ("SP"=w281:u8[])
        n140 = Build Array(w266, w267) -> (w268:u8[])
        n141 = Multiply(x=100000.0, y=w248) -> (x*y=w274:dbl)
        n142 = Reverse 1D Array(array=w272) -> (reversed array=w263:u8[])
        n143 = call "DoubleToSetpoint.vi"("Double"=w274) -> ("SP"=w261:u8[])
        n144 = Reverse 1D Array(array=w268) -> (reversed array=w262:u8[])
        n145 = Build Array (concatenate)(w282, w281) -> (w284:u8[])
        n146 = Build Array (concatenate)(w263, w262, w261) -> (w259:u8[])
        n147 = Bundle By Name(cluster=T3 {"timestamp"=timestamp(0 s since 1904-01-01), "payload"=[], "identifier"=0, "type"=0, "extended?"=FALSE, "echo?"=FALSE} ("CAN frame 3"), "payload"=w259, "identifier"=u32 20) -> (w256:T3)
        n148 = Bundle By Name(cluster=T3 {"timestamp"=timestamp(0 s since 1904-01-01), "payload"=[], "identifier"=0, "type"=0, "extended?"=FALSE, "echo?"=FALSE} ("CAN frame 3"), "payload"=w284, "identifier"=u32 19) -> (w257:T3)
        n149 = Build Array(w256, w257) -> (w255:T3[])
        n150 = Build Array(w256) -> ()  [unwired: 1 out]
        n151 = local read "Ready 1"() -> (w286:bool)
        n152 = local read "ON 1"() -> (w287:bool)
        n153 = Or(x=w287, y=w286) -> (x .or. y?=w288:bool)
      }
      frame 5 {
        n154 = local write "To ACT CH 1"(FALSE ("Idc cmd")) -> ()
        n155 = local write "SEND sp 1"(TRUE ("SEND sp 1")) -> ()
        n156 = Replace Array Subset(array=w299, new element=u8 1 ("new element/subarray"), index=0) -> (w291:u8[])
        n157 = Bundle By Name(cluster=T3 {"timestamp"=timestamp(0 s since 1904-01-01), "payload"=[], "identifier"=0, "type"=0, "extended?"=FALSE, "echo?"=FALSE} ("CAN frame 3"), "payload"=w291, "identifier"=u32 24) -> (w293:T3)
        n158 = Build Array(w293) -> (w292:T3[])
      }
      frame 6 {
        n159 = local write "Clear 2"(FALSE ("Clear")) -> ()
        n160 = Replace Array Subset(array=w309, new element=u8 40 ("new element/subarray"), index=1) -> (w303:u8[])
        n161 = Bundle By Name(cluster=T3 {"timestamp"=timestamp(0 s since 1904-01-01), "payload"=[], "identifier"=0, "type"=0, "extended?"=FALSE, "echo?"=FALSE} ("CAN frame 3"), "payload"=w303, "identifier"=u32 40) -> (w304:T3)
        n162 = Build Array(w304) -> (w301:T3[])
      }
      frame 7 {
        n163 = local write "Shutdwn 2"(FALSE ("Shutdwn")) -> ()
        n164 = Replace Array Subset(array=w319, new element=u8 20 ("new element/subarray"), index=0) -> (w313:u8[])
        n165 = Bundle By Name(cluster=T3 {"timestamp"=timestamp(0 s since 1904-01-01), "payload"=[], "identifier"=0, "type"=0, "extended?"=FALSE, "echo?"=FALSE} ("CAN frame 3"), "payload"=w313, "identifier"=u32 40) -> (w314:T3)
        n166 = Build Array(w314) -> (w312:T3[])
      }
      frame 8 {
        n167 = local write "Emergency 2"(FALSE ("Idc cmd")) -> ()
        n168 = Replace Array Subset(array=w329, new element=u8 30 ("new element/subarray"), index=0) -> (w323:u8[])
        n169 = Bundle By Name(cluster=T3 {"timestamp"=timestamp(0 s since 1904-01-01), "payload"=[], "identifier"=0, "type"=0, "extended?"=FALSE, "echo?"=FALSE} ("CAN frame 3"), "payload"=w323, "identifier"=u32 40) -> (w324:T3)
        n170 = Build Array(w324) -> (w321:T3[])
      }
      frame 9 {
        n171 = local write "SEND sp 2"(TRUE ("SEND sp 2")) -> ()
        n172 = local write "To IN OP  2"(FALSE ("Idc cmd")) -> ()
        n173 = Replace Array Subset(array=w340, new element=u8 2 ("new element/subarray"), index=0) -> (w334:u8[])
        n174 = Bundle By Name(cluster=T3 {"timestamp"=timestamp(0 s since 1904-01-01), "payload"=[], "identifier"=0, "type"=0, "extended?"=FALSE, "echo?"=FALSE} ("CAN frame 3"), "payload"=w334, "identifier"=u32 40) -> (w335:T3)
        n175 = Build Array(w335) -> (w332:T3[])
      }
      frame 10 {
        # "Vdc Q mode"
        n176 = Unbundle By Name(w345) -> ("IC2_P_gain"=w346:dbl)
        n177 = Unbundle By Name(w345) -> ("IC2_P_bias"=w347:dbl)
        n178 = Unbundle By Name(w345) -> ("IC2_Q_gain"=w349:dbl)
        n179 = Unbundle By Name(w345) -> ("IC2_Q_bias"=w348:dbl)
        n180 = Multiply(x=w346, y="Pac2") -> (x*y=w355:dbl)
        n181 = Multiply(x=w349, y="Qac2") -> (x*y=w354:dbl)
        n182 = Add(x=w354, y=w348) -> (x+y=w351:dbl)
        n183 = Add(x=w355, y=w347) -> (x+y=w344:dbl)
        n184 = Add(x=w351, y="Q2 bias") -> (x+y=w350:dbl)
        n185 = Add(x="P2 bias", y=w344) -> (x+y=w343:dbl)
        n186 = call "Q_limiter.vi"("IN Q"=w343) -> ("OUT Q"=w357:dbl)  [unwired: 10 in]
        n187 = call "Q_limiter.vi"("IN Q"=w350) -> ("OUT Q"=w359:dbl)  [unwired: 10 in]
        n188 = call "DoubleToSetpoint.vi"("Double"=w357) -> ("SP"=w361:u8[])
        n189 = call "DoubleToSetpoint.vi"("Double"=w359) -> ("SP"=w360:u8[])
        n190 = Build Array (concatenate)(w361, w360) -> (w364:u8[])
        n191 = local write "SEND sp 2"(FALSE ("SEND sp 2")) -> ()
        n192 = Bundle By Name(cluster=T3 {"timestamp"=timestamp(0 s since 1904-01-01), "payload"=[], "identifier"=0, "type"=0, "extended?"=FALSE, "echo?"=FALSE} ("CAN frame 3"), "payload"=w364, "identifier"=u32 35) -> (w365:T3)
        n193 = Build Array(w365) -> (w362:T3[])
        n194 = local read "ON 2"() -> (w368:bool)
        n195 = local read "Ready 2"() -> (w369:bool)
        n196 = Or(x=w368, y=w369) -> (x .or. y?=w367:bool)
      }
      frame 11 {
        n197 = local write "To ACT CH 2"(FALSE ("Idc cmd")) -> ()
        n198 = local write "SEND sp 2"(TRUE ("SEND sp 2")) -> ()
        n199 = Replace Array Subset(array=w379, new element=u8 1 ("new element/subarray"), index=0) -> (w371:u8[])
        n200 = Bundle By Name(cluster=T3 {"timestamp"=timestamp(0 s since 1904-01-01), "payload"=[], "identifier"=0, "type"=0, "extended?"=FALSE, "echo?"=FALSE} ("CAN frame 3"), "payload"=w371, "identifier"=u32 40) -> (w373:T3)
        n201 = Build Array(w373) -> (w372:T3[])
      }
      frame 12 {
        n202 = local write "Clear 3"(FALSE ("Clear")) -> ()
        n203 = Replace Array Subset(array=w389, new element=u8 40 ("new element/subarray"), index=1) -> (w383:u8[])
        n204 = Bundle By Name(cluster=T3 {"timestamp"=timestamp(0 s since 1904-01-01), "payload"=[], "identifier"=0, "type"=0, "extended?"=FALSE, "echo?"=FALSE} ("CAN frame 3"), "payload"=w383, "identifier"=u32 56) -> (w384:T3)
        n205 = Build Array(w384) -> (w381:T3[])
      }
      frame 13 {
        n206 = local write "Shutdwn 3"(FALSE ("Shutdwn")) -> ()
        n207 = Replace Array Subset(array=w399, new element=u8 20 ("new element/subarray"), index=0) -> (w393:u8[])
        n208 = Bundle By Name(cluster=T3 {"timestamp"=timestamp(0 s since 1904-01-01), "payload"=[], "identifier"=0, "type"=0, "extended?"=FALSE, "echo?"=FALSE} ("CAN frame 3"), "payload"=w393, "identifier"=u32 56) -> (w394:T3)
        n209 = Build Array(w394) -> (w391:T3[])
      }
      frame 14 {
        n210 = local write "Emergency 3"(FALSE ("Idc cmd")) -> ()
        n211 = Replace Array Subset(array=w409, new element=u8 30 ("new element/subarray"), index=0) -> (w403:u8[])
        n212 = Bundle By Name(cluster=T3 {"timestamp"=timestamp(0 s since 1904-01-01), "payload"=[], "identifier"=0, "type"=0, "extended?"=FALSE, "echo?"=FALSE} ("CAN frame 3"), "payload"=w403, "identifier"=u32 56) -> (w404:T3)
        n213 = Build Array(w404) -> (w401:T3[])
      }
      frame 15 {
        n214 = local write "SEND sp 3"(TRUE ("SEND sp 3")) -> ()
        n215 = local write "To IN OP  3"(FALSE ("Idc cmd")) -> ()
        n216 = Replace Array Subset(array=w420, new element=u8 2 ("new element/subarray"), index=0) -> (w414:u8[])
        n217 = Bundle By Name(cluster=T3 {"timestamp"=timestamp(0 s since 1904-01-01), "payload"=[], "identifier"=0, "type"=0, "extended?"=FALSE, "echo?"=FALSE} ("CAN frame 3"), "payload"=w414, "identifier"=u32 56) -> (w415:T3)
        n218 = Build Array(w415) -> (w412:T3[])
      }
      frame 16 {
        # "Vdc Q mode"
        n219 = Unbundle By Name(w422) -> ("IC3_P_gain"=w424:dbl)
        n220 = Unbundle By Name(w422) -> ("IC3_Q_gain"=w426:dbl)
        n221 = Unbundle By Name(w422) -> ("IC3_Q_bias"=w425:dbl)
        n222 = Unbundle By Name(w422) -> ("IC3_P_bias"=w423:dbl)
        n223 = Multiply(x=w424, y="Pac3") -> (x*y=w432:dbl)
        n224 = Multiply(x=w426, y="Qac3") -> (x*y=w431:dbl)
        n225 = local write "SEND sp 3"(FALSE ("SEND sp")) -> ()
        n226 = Add(x=w432, y=w423) -> (x+y=w428:dbl)
        n227 = Add(x=w431, y=w425) -> (x+y=w427:dbl)
        n228 = call "Q_limiter.vi"("IN Q"=w428) -> ("OUT Q"=w433:dbl)  [unwired: 10 in]
        n229 = call "Q_limiter.vi"("IN Q"=w427) -> ("OUT Q"=w434:dbl)  [unwired: 10 in]
        n230 = call "DoubleToSetpoint.vi"("Double"=w433) -> ("SP"=w436:u8[])
        n231 = call "DoubleToSetpoint.vi"("Double"=w434) -> ("SP"=w435:u8[])
        n232 = Build Array (concatenate)(w436, w435) -> (w439:u8[])
        n233 = local read "ON 3"() -> (w444:bool)
        n234 = local read "Ready 3"() -> (w442:bool)
        n235 = Or(x=w444, y=w442) -> (x .or. y?=w443:bool)
        n236 = Bundle By Name(cluster=T3 {"timestamp"=timestamp(0 s since 1904-01-01), "payload"=[], "identifier"=0, "type"=0, "extended?"=FALSE, "echo?"=FALSE} ("CAN frame 3"), "payload"=w439, "identifier"=u32 51) -> (w440:T3)
        n237 = Build Array(w440) -> (w437:T3[])
      }
      frame 17 {
        n238 = local write "To ACT CH 3"(FALSE ("Idc cmd")) -> ()
        n239 = local write "SEND sp 3"(TRUE ("SEND sp 3")) -> ()
        n240 = Replace Array Subset(array=w455, new element=u8 1 ("new element/subarray"), index=0) -> (w448:u8[])
        n241 = Bundle By Name(cluster=T3 {"timestamp"=timestamp(0 s since 1904-01-01), "payload"=[], "identifier"=0, "type"=0, "extended?"=FALSE, "echo?"=FALSE} ("CAN frame 3"), "payload"=w448, "identifier"=u32 56) -> (w449:T3)
        n242 = Build Array(w449) -> (w446:T3[])
      }
      frame 18 {
        n243 = local write "Clear 4"(FALSE ("Clear")) -> ()
        n244 = Replace Array Subset(array=w465, new element=u8 40 ("new element/subarray"), index=1) -> (w458:u8[])
        n245 = Bundle By Name(cluster=T3 {"timestamp"=timestamp(0 s since 1904-01-01), "payload"=[], "identifier"=0, "type"=0, "extended?"=FALSE, "echo?"=FALSE} ("CAN frame 3"), "payload"=w458, "identifier"=u32 72) -> (w460:T3)
        n246 = Build Array(w460) -> (w459:T3[])
      }
      frame 19 {
        n247 = local write "Shutdwn 4"(FALSE ("Shutdwn")) -> ()
        n248 = Replace Array Subset(array=w475, new element=u8 20 ("new element/subarray"), index=0) -> (w468:u8[])
        n249 = Bundle By Name(cluster=T3 {"timestamp"=timestamp(0 s since 1904-01-01), "payload"=[], "identifier"=0, "type"=0, "extended?"=FALSE, "echo?"=FALSE} ("CAN frame 3"), "payload"=w468, "identifier"=u32 72) -> (w470:T3)
        n250 = Build Array(w470) -> (w469:T3[])
      }
      frame 20 {
        n251 = local write "Emergency 4"(FALSE ("Idc cmd")) -> ()
        n252 = Replace Array Subset(array=w485, new element=u8 30 ("new element/subarray"), index=0) -> (w478:u8[])
        n253 = Bundle By Name(cluster=T3 {"timestamp"=timestamp(0 s since 1904-01-01), "payload"=[], "identifier"=0, "type"=0, "extended?"=FALSE, "echo?"=FALSE} ("CAN frame 3"), "payload"=w478, "identifier"=u32 72) -> (w480:T3)
        n254 = Build Array(w480) -> (w479:T3[])
      }
      frame 21 {
        n255 = local write "SEND sp 4"(TRUE ("SEND sp 4")) -> ()
        n256 = local write "To IN OP  4"(FALSE ("Idc cmd")) -> ()
        n257 = Replace Array Subset(array=w496, new element=u8 2 ("new element/subarray"), index=0) -> (w490:u8[])
        n258 = Bundle By Name(cluster=T3 {"timestamp"=timestamp(0 s since 1904-01-01), "payload"=[], "identifier"=0, "type"=0, "extended?"=FALSE, "echo?"=FALSE} ("CAN frame 3"), "payload"=w490, "identifier"=u32 72) -> (w491:T3)
        n259 = Build Array(w491) -> (w488:T3[])
      }
      frame 22 {
        # "Vdc Q mode"
        n260 = Add(x="Qac4", y="biasQ4") -> (x+y=w498:dbl)
        n261 = local write "SEND sp 4"(FALSE ("SEND sp")) -> ()
        n262 = Add(x="Vdc4", y="biasV4") -> (x+y=w502:dbl)
        n263 = call "Q_limiter.vi"("IN Q"=w498) -> ("OUT Q"=w504:dbl)  [unwired: 10 in]
        n264 = call "Vdc_lim.vi"("IN Vdc"=w502) -> ("OUT Vdc"=w505:dbl)  [unwired: 10 in]
        n265 = call "DoubleToSetpoint.vi"("Double"=w505) -> ("SP"=w507:u8[])
        n266 = call "DoubleToSetpoint.vi"("Double"=w504) -> ("SP"=w506:u8[])
        n267 = Build Array (concatenate)(w507, w506) -> (w510:u8[])
        n268 = local read "ON 4"() -> (w514:bool)
        n269 = local read "Ready 4"() -> (w515:bool)
        n270 = Or(x=w514, y=w515) -> (x .or. y?=w513:bool)
        n271 = Bundle By Name(cluster=T3 {"timestamp"=timestamp(0 s since 1904-01-01), "payload"=[], "identifier"=0, "type"=0, "extended?"=FALSE, "echo?"=FALSE} ("CAN frame 3"), "payload"=w510, "identifier"=u32 67) -> (w511:T3)
        n272 = Build Array(w511) -> (w508:T3[])
      }
      frame 23 {
        n273 = local write "To ACT CH 4"(FALSE ("Idc cmd")) -> ()
        n274 = local write "SEND sp 4"(TRUE ("SEND sp 4")) -> ()
        n275 = Replace Array Subset(array=w526, new element=u8 1 ("new element/subarray"), index=0) -> (w519:u8[])
        n276 = Bundle By Name(cluster=T3 {"timestamp"=timestamp(0 s since 1904-01-01), "payload"=[], "identifier"=0, "type"=0, "extended?"=FALSE, "echo?"=FALSE} ("CAN frame 3"), "payload"=w519, "identifier"=u32 72) -> (w520:T3)
        n277 = Build Array(w520) -> (w517:T3[])
      }
      frame 24 {
        # "it take on average 500ms to close the switch\n-> therefore, we wait 200ms so the converter is only following in grid connected mode for 300ms\n-> this guarentees a more smooth stransition"
        # "start forming 1"
        n278 = local write "Start forming 1"(FALSE ("Start following 1")) -> ()
        n279 = local write "SEND sp 1"(TRUE ("SEND sp 1")) -> ()
        n280 = Replace Array Subset(array=w538, new element=u8 3 ("new element/subarray"), index=0) -> (w533:u8[])
        n281 = flat-sequence {
          tunnel: [TRUE] -> w528
          tunnel: [w542] -> w529
          tunnel: w528 -> [w542]
          frame #0 {
          }
          frame #1 {
            # "40"
            n282 = Wait (ms)(milliseconds to wait=u32 80) -> ()  [unwired: 1 out]
          }
        }
        n283 = Bundle By Name(cluster=T3 {"timestamp"=timestamp(0 s since 1904-01-01), "payload"=[], "identifier"=0, "type"=0, "extended?"=FALSE, "echo?"=FALSE} ("CAN frame 3"), "payload"=w533, "identifier"=u32 24) -> (w534:T3)
        n284 = Build Array(w534) -> (w531:T3[])
      }
      frame 25 {
        # "it take on average 140ms to open the switch\n-> to be sure the grid is connected before we stors following, we add a 300ms delay\n-> the converter can easily sustain 160ms in forming mode when grid connected"
        # "start following 1"
        n285 = local write "Start following 1"(FALSE ("Start forming 1")) -> ()
        n286 = local write "SEND sp 1"(TRUE ("SEND sp 1")) -> ()
        n287 = Replace Array Subset(array=w552, new element=u8 2 ("new element/subarray"), index=0) -> (w546:u8[])
        n288 = Bundle By Name(cluster=T3 {"timestamp"=timestamp(0 s since 1904-01-01), "payload"=[], "identifier"=0, "type"=0, "extended?"=FALSE, "echo?"=FALSE} ("CAN frame 3"), "payload"=w546, "identifier"=u32 24) -> (w547:T3)
        n289 = Build Array(w547) -> (w544:T3[])
      }
      frame 99, Default {
        n290 = Bundle By Name(cluster=T3 {"timestamp"=timestamp(0 s since 1904-01-01), "payload"=[], "identifier"=0, "type"=0, "extended?"=FALSE, "echo?"=FALSE} ("CAN frame 3"), "payload"=w554, "identifier"=u32 18) -> (w557:T3)
        n291 = Build Array(w557) -> (w556:T3[])
      }
    }
    n292 = case shown="True" w153 {
      tunnel: w152 -> [w194 _]
      tunnel: w188 -> [w196 _]
      tunnel: [w195 _] -> w187
      frame True {
        n293 = call-poly <vilib>:"XNET Write.vi"("session in"=w196, "data"=w194) -> ("session out"=w195:refnum<k21>)  [unwired: 12 in, 1 out]
        "CAN OUT" <- w194
      }
      frame False {
      }
    }
    n294 = node-c288() -> ()  [unwired: 1 in, 1 out]
  }
  n295 = timed-loop {
    timing: w35 -> [_]
    timing-out: [_] -> w34
    tunnel: w33 -> [w563]
    tunnel: [w569] -> w40
    shift-right: [w564] -> _
    shift-left: T7 {"State 1"=4.0, "code 1"=0.0, "code 2"=0.0, "code 3"=0.0, "code 4"=0.0, "State 2"=4.0, "State 3"=4.0, "State 4"=4.0} ("Conv 2") -> [w568]
    tunnel: [FALSE ("stop CAN")] -> w37
    shift-right: [w561] -> _
    shift-left: T5 {"Vdc1"=0.0, "P1"=0.0, "Vdc2"=0.0, "P2"=0.0, "Q2"=0.0, "Vdc3"=0.0, "P3"=0.0, "Q3"=0.0, "Vdc4"=0.0, "P4"=0.0, "Q4"=0.0, "Q1"=0.0} ("measurements 2") -> [w562]
    stop <- w567 stop-if-true
    # "state 21: forming, state 23 is following"
    # "READ CAN FROM CONVERTER"
    n296 = node-c288() -> ()  [unwired: 1 in, 1 out]
    n297 = local write "CAN with Conv"(TRUE) -> ()
    n298 = call-poly <vilib>:"XNET Read.vi"("session in"=w563) -> ("session out"=w569:refnum<k21>, "data"=w570:T3[])  [unwired: 11 in, 2 out]
    n299 = Get Date/Time In Seconds() -> (seconds since 1Jan1904=→"current time":timestamp)
    n300 = for {
      tunnel: w570 -> [w575] mode=indexing
      shift-right: [w573] -> w564
      shift-left: w568 -> [w574]
      shift-right: [w571] -> w561
      shift-left: w562 -> [w572]
      n301 = Unbundle By Name(w575) -> ("identifier"=w577:u32, "payload"=w576:u8[])
      n302 = case shown="206" w577 {
        tunnel: w576 -> [_ w584 w618 w643 w668 w695 w702 w709 w716 w721 w729 w737 w745]
        tunnel: w574 -> [w579 w592 w626 w651 w676 w693 w700 w707 w714 w719 w725 w734 w742]
        tunnel: [w579 w591 w625 w650 w675 w693 w700 w707 w714 w719 w725 w734 w742] -> w573
        tunnel: w572 -> [w578 w581 w615 w640 w666 w691 w696 w703 w710 w717 w724 w733 w740]
        tunnel: [w578 w582 w616 w641 w667 w692 w697 w704 w711 w718 w723 w732 w741] -> w571
        frame 0, Default {
        }
        frame 25 {
          w580 = 1.0 ("factor 1")
          n303 = Index Array(array=w584, index=0) -> (element=w585:u8)
          n304 = call "U8arrayToMeasurement.vi"("factor 2"=w580, "factor 1"=w580, "payload"=w584) -> ("Meas 2"=w583:dbl)  [unwired: 1 out]
          "V slider 19" <- w583
          n305 = Index Array(array=w584, index=1) -> (element=w588:u8)
          n306 = Index Array(array=w584, index=2) -> (element=w587:u8)
          n307 = Join Numbers(hi=w588, lo=w587) -> ((hi.lo)=w586:u16)
          "State code 1" <- w586
          n308 = Bundle By Name(cluster=w581, "Vdc1"=w583) -> (w582:T5)
          n309 = case shown="5" w585 {
            frame 5 {
              w595 = FALSE ("Fault 1")
              n310 = local write "Forming 1"(FALSE ("Forming 1")) -> ()
              n311 = local write "Fault 1"(TRUE ("Fault 1")) -> ()
              n312 = local write "Error 1"(w595) -> ()
              n313 = local write "OFF 1"(w595) -> ()
              n314 = local write "Ready 1"(w595) -> ()
              n315 = local write "ON 1"(w595) -> ()
            }
            frame 6 {
              w599 = FALSE ("Fault 1")
              n316 = local write "Fault 1"(w599) -> ()
              n317 = local write "Error 1"(w599) -> ()
              n318 = local write "OFF 1"(w599) -> ()
              n319 = local write "Ready 1"(w599) -> ()
              n320 = local write "ON 1"(TRUE ("Fault 1")) -> ()
              n321 = local write "Forming 1"(TRUE ("Forming 1")) -> ()
            }
            frame 1 {
              w601 = FALSE ("Fault 1")
              n322 = local write "Forming 1"(FALSE ("Forming 1")) -> ()
              n323 = local write "Fault 1"(w601) -> ()
              n324 = local write "Error 1"(TRUE ("Error 1")) -> ()
              n325 = local write "OFF 1"(w601) -> ()
              n326 = local write "Ready 1"(w601) -> ()
              n327 = local write "ON 1"(w601) -> ()
            }
            frame 2 {
              w605 = FALSE ("Fault 1")
              n328 = local write "Forming 1"(FALSE ("Forming 1")) -> ()
              n329 = local write "Fault 1"(w605) -> ()
              n330 = local write "Error 1"(w605) -> ()
              n331 = local write "OFF 1"(TRUE ("OFF 1")) -> ()
              n332 = local write "Ready 1"(w605) -> ()
              n333 = local write "ON 1"(w605) -> ()
            }
            frame 3 {
              w608 = FALSE ("Fault 1")
              n334 = local write "Forming 1"(FALSE ("Forming 1")) -> ()
              n335 = local write "Fault 1"(w608) -> ()
              n336 = local write "Error 1"(w608) -> ()
              n337 = local write "OFF 1"(w608) -> ()
              n338 = local write "Ready 1"(TRUE ("Ready 1")) -> ()
              n339 = local write "ON 1"(w608) -> ()
            }
            frame 4 {
              w611 = FALSE ("Fault 1")
              n340 = local write "Fault 1"(w611) -> ()
              n341 = local write "Error 1"(w611) -> ()
              n342 = local write "OFF 1"(w611) -> ()
              n343 = local write "Ready 1"(w611) -> ()
              n344 = local write "Forming 1"(FALSE ("Forming 1")) -> ()
              n345 = local write "ON 1"(TRUE ("ON 1")) -> ()
            }
            frame 99, Default {
              w613 = FALSE ("Fault 1")
              n346 = local write "Forming 1"(FALSE ("Forming 1")) -> ()
              n347 = local write "Fault 1"(w613) -> ()
              n348 = local write "Error 1"(w613) -> ()
              n349 = local write "OFF 1"(w613) -> ()
              n350 = local write "Ready 1"(w613) -> ()
              n351 = local write "ON 1"(w613) -> ()
            }
          }
          n352 = Bundle By Name(cluster=w592, "State 1"=w585, "code 1"=w586) -> (w591:T7)
        }
        frame 41 {
          w614 = 1.0 ("factor 1")
          n353 = call "U8arrayToMeasurement.vi"("factor 2"=w614, "factor 1"=w614, "payload"=w618) -> ("Meas 2"=w617:dbl)  [unwired: 1 out]
          "V slider 20" <- w617
          n354 = Index Array(array=w618, index=0) -> (element=w624:u8)
          n355 = Index Array(array=w618, index=1) -> (element=w621:u8)
          n356 = Index Array(array=w618, index=2) -> (element=w620:u8)
          n357 = Join Numbers(hi=w621, lo=w620) -> ((hi.lo)=w619:u16)
          "State code 2" <- w619
          n358 = Bundle By Name(cluster=w615, "Vdc2"=w617) -> (w616:T5)
          n359 = case shown="5" w624 {
            frame 5 {
              w629 = FALSE ("Fault 1")
              n360 = local write "Fault 2"(TRUE ("Fault 1")) -> ()
              n361 = local write "Error 2"(w629) -> ()
              n362 = local write "OFF 2"(w629) -> ()
              n363 = local write "Ready 2"(w629) -> ()
              n364 = local write "ON 2"(w629) -> ()
            }
            frame 1 {
              w630 = FALSE ("Fault 1")
              n365 = local write "Fault 2"(w630) -> ()
              n366 = local write "Error 2"(TRUE ("Error 1")) -> ()
              n367 = local write "OFF 2"(w630) -> ()
              n368 = local write "Ready 2"(w630) -> ()
              n369 = local write "ON 2"(w630) -> ()
            }
            frame 2 {
              w633 = FALSE ("Fault 1")
              n370 = local write "Fault 2"(w633) -> ()
              n371 = local write "Error 2"(w633) -> ()
              n372 = local write "OFF 2"(TRUE ("OFF 1")) -> ()
              n373 = local write "Ready 2"(w633) -> ()
              n374 = local write "ON 2"(w633) -> ()
            }
            frame 3 {
              w635 = FALSE ("Fault 1")
              n375 = local write "Fault 2"(w635) -> ()
              n376 = local write "Error 2"(w635) -> ()
              n377 = local write "OFF 2"(w635) -> ()
              n378 = local write "Ready 2"(TRUE ("Ready 1")) -> ()
              n379 = local write "ON 2"(w635) -> ()
            }
            frame 4 {
              w637 = FALSE ("Fault 1")
              n380 = local write "Fault 2"(w637) -> ()
              n381 = local write "Error 2"(w637) -> ()
              n382 = local write "OFF 2"(w637) -> ()
              n383 = local write "Ready 2"(w637) -> ()
              n384 = local write "ON 2"(TRUE ("ON 1")) -> ()
            }
            frame 99, Default {
              w638 = FALSE ("Fault 1")
              n385 = local write "Fault 2"(w638) -> ()
              n386 = local write "Error 2"(w638) -> ()
              n387 = local write "OFF 2"(w638) -> ()
              n388 = local write "Ready 2"(w638) -> ()
              n389 = local write "ON 2"(w638) -> ()
            }
          }
          n390 = Bundle By Name(cluster=w626, "State 2"=w624, "code 2"=w619) -> (w625:T7)
        }
        frame 57 {
          w639 = 1.0 ("factor 1")
          n391 = Index Array(array=w643, index=0) -> (element=w649:u8)
          n392 = Index Array(array=w643, index=1) -> (element=w646:u8)
          n393 = Index Array(array=w643, index=2) -> (element=w645:u8)
          n394 = call "U8arrayToMeasurement.vi"("factor 2"=w639, "factor 1"=w639, "payload"=w643) -> ("Meas 2"=w642:dbl)  [unwired: 1 out]
          "V slider 21" <- w642
          n395 = Join Numbers(hi=w646, lo=w645) -> ((hi.lo)=w644:u16)
          "State code 3" <- w644
          n396 = case shown="5" w649 {
            frame 5 {
              w654 = FALSE ("Fault 1")
              n397 = local write "Fault 3"(TRUE ("Fault 1")) -> ()
              n398 = local write "Error 3"(w654) -> ()
              n399 = local write "OFF 3"(w654) -> ()
              n400 = local write "Ready 3"(w654) -> ()
              n401 = local write "ON 3"(w654) -> ()
            }
            frame 1 {
              w655 = FALSE ("Fault 1")
              n402 = local write "Fault 3"(w655) -> ()
              n403 = local write "Error 3"(TRUE ("Error 1")) -> ()
              n404 = local write "OFF 3"(w655) -> ()
              n405 = local write "Ready 3"(w655) -> ()
              n406 = local write "ON 3"(w655) -> ()
            }
            frame 2 {
              w658 = FALSE ("Fault 1")
              n407 = local write "Fault 3"(w658) -> ()
              n408 = local write "Error 3"(w658) -> ()
              n409 = local write "OFF 3"(TRUE ("OFF 1")) -> ()
              n410 = local write "Ready 3"(w658) -> ()
              n411 = local write "ON 3"(w658) -> ()
            }
            frame 3 {
              w660 = FALSE ("Fault 1")
              n412 = local write "Fault 3"(w660) -> ()
              n413 = local write "Error 3"(w660) -> ()
              n414 = local write "OFF 3"(w660) -> ()
              n415 = local write "Ready 3"(TRUE ("Ready 1")) -> ()
              n416 = local write "ON 3"(w660) -> ()
            }
            frame 4 {
              w662 = FALSE ("Fault 1")
              n417 = local write "Fault 3"(w662) -> ()
              n418 = local write "Error 3"(w662) -> ()
              n419 = local write "OFF 3"(w662) -> ()
              n420 = local write "Ready 3"(w662) -> ()
              n421 = local write "ON 3"(TRUE ("ON 1")) -> ()
            }
            frame 99, Default {
              w663 = FALSE ("Fault 1")
              n422 = local write "Fault 3"(w663) -> ()
              n423 = local write "Error 3"(w663) -> ()
              n424 = local write "OFF 3"(w663) -> ()
              n425 = local write "Ready 3"(w663) -> ()
              n426 = local write "ON 3"(w663) -> ()
            }
          }
          n427 = Bundle By Name(cluster=w640, "Vdc3"=w642) -> (w641:T5)
          n428 = Bundle By Name(cluster=w651, "State 3"=w649, "code 3"=w644) -> (w650:T7)
        }
        frame 73 {
          w664 = 1.0 ("factor 1")
          n429 = Index Array(array=w668, index=0) -> (element=w674:u8)
          n430 = Index Array(array=w668, index=1) -> (element=w671:u8)
          n431 = Index Array(array=w668, index=2) -> (element=w670:u8)
          n432 = Join Numbers(hi=w671, lo=w670) -> ((hi.lo)=w669:u16)
          "State code 4" <- w669
          n433 = call "U8arrayToMeasurement.vi"("factor 2"=w664, "factor 1"=w664, "payload"=w668) -> ("Meas 2"=w665:dbl)  [unwired: 1 out]
          "V slider 22" <- w665
          n434 = case shown="5" w674 {
            frame 5 {
              w679 = FALSE ("Fault 1")
              n435 = local write "Fault 4"(TRUE ("Fault 1")) -> ()
              n436 = local write "Error 4"(w679) -> ()
              n437 = local write "OFF 4"(w679) -> ()
              n438 = local write "Ready 4"(w679) -> ()
              n439 = local write "ON 4"(w679) -> ()
            }
            frame 1 {
              w680 = FALSE ("Fault 1")
              n440 = local write "Fault 4"(w680) -> ()
              n441 = local write "Error 4"(TRUE ("Error 1")) -> ()
              n442 = local write "OFF 4"(w680) -> ()
              n443 = local write "Ready 4"(w680) -> ()
              n444 = local write "ON 4"(w680) -> ()
            }
            frame 2 {
              w683 = FALSE ("Fault 1")
              n445 = local write "Fault 4"(w683) -> ()
              n446 = local write "Error 4"(w683) -> ()
              n447 = local write "OFF 4"(TRUE ("OFF 1")) -> ()
              n448 = local write "Ready 4"(w683) -> ()
              n449 = local write "ON 4"(w683) -> ()
            }
            frame 3 {
              w685 = FALSE ("Fault 1")
              n450 = local write "Fault 4"(w685) -> ()
              n451 = local write "Error 4"(w685) -> ()
              n452 = local write "OFF 4"(w685) -> ()
              n453 = local write "Ready 4"(TRUE ("Ready 1")) -> ()
              n454 = local write "ON 4"(w685) -> ()
            }
            frame 4 {
              w687 = FALSE ("Fault 1")
              n455 = local write "Fault 4"(w687) -> ()
              n456 = local write "Error 4"(w687) -> ()
              n457 = local write "OFF 4"(w687) -> ()
              n458 = local write "Ready 4"(w687) -> ()
              n459 = local write "ON 4"(TRUE ("ON 1")) -> ()
            }
            frame 99, Default {
              w688 = FALSE ("Fault 1")
              n460 = local write "Fault 4"(w688) -> ()
              n461 = local write "Error 4"(w688) -> ()
              n462 = local write "OFF 4"(w688) -> ()
              n463 = local write "Ready 4"(w688) -> ()
              n464 = local write "ON 4"(w688) -> ()
            }
          }
          n465 = Bundle By Name(cluster=w666, "Vdc4"=w665) -> (w667:T5)
          n466 = Bundle By Name(cluster=w676, "State 4"=w674, "code 4"=w669) -> (w675:T7)
        }
        frame 258 {
          w694 = 1000.0 ("factor 1")
          # "Q"
          # "P"
          n467 = call "U8arrayToMeasurement.vi"("factor 2"=w694, "factor 1"=w694, "payload"=w695) -> ("Meas 2"=w689:dbl, "Meas 1"=w690:dbl)
          "kW" <- w690
          "?VkVAr" <- w689
          n468 = Bundle By Name(cluster=w691, "P1"=w690, "Q1"=w689) -> (w692:T5)
        }
        frame 514 {
          w701 = 1000.0 ("factor 1")
          # "Q"
          # "P"
          n469 = call "U8arrayToMeasurement.vi"("factor 2"=w701, "factor 1"=w701, "payload"=w702) -> ("Meas 2"=w698:dbl, "Meas 1"=w699:dbl)
          "kW" <- w699
          "?VkVAr" <- w698
          n470 = Bundle By Name(cluster=w696, "P2"=w699, "Q2"=w698) -> (w697:T5)
        }
        frame 770 {
          w708 = 1000.0 ("factor 1")
          # "Q"
          # "P"
          n471 = call "U8arrayToMeasurement.vi"("factor 2"=w708, "factor 1"=w708, "payload"=w709) -> ("Meas 2"=w705:dbl, "Meas 1"=w706:dbl)
          "kW" <- w706
          "?VkVAr" <- w705
          n472 = Bundle By Name(cluster=w703, "P3"=w706, "Q3"=w705) -> (w704:T5)
        }
        frame 1026 {
          w715 = 1000.0 ("factor 1")
          # "Q"
          # "P"
          n473 = call "U8arrayToMeasurement.vi"("factor 2"=w715, "factor 1"=w715, "payload"=w716) -> ("Meas 2"=w712:dbl, "Meas 1"=w713:dbl)
          "kW" <- w713
          "?VkVAr" <- w712
          n474 = Bundle By Name(cluster=w710, "P4"=w713, "Q4"=w712) -> (w711:T5)
        }
        frame 262 {
          w722 = 1.0 ("factor 1")
          n475 = call "U8arrayToMeasurement.vi"("factor 2"=w722, "factor 1"=w722, "payload"=w721) -> ("Meas 1"=w720:dbl)  [unwired: 1 out]
          n476 = Bundle By Name(cluster=w717, "Vdc1"=w720) -> (w718:T5)
        }
        frame 518 {
          w730 = 1.0 ("factor 1")
          # "Vdc"
          n477 = call "U8arrayToMeasurement.vi"("factor 2"=w730, "factor 1"=w730, "payload"=w729) -> ("Meas 2"=w727:dbl, "Meas 1"=w728:dbl)
          n478 = Add(x=w728, y=w727) -> (x+y=w726:dbl)
          n479 = Bundle By Name(cluster=w724, "Vdc2"=w726) -> (w723:T5)
        }
        frame 774 {
          w738 = 1.0 ("factor 1")
          # "Vdc"
          n480 = call "U8arrayToMeasurement.vi"("factor 2"=w738, "factor 1"=w738, "payload"=w737) -> ("Meas 2"=w735:dbl, "Meas 1"=w736:dbl)
          n481 = Add(x=w736, y=w735) -> (x+y=w731:dbl)
          n482 = Bundle By Name(cluster=w733, "Vdc3"=w731) -> (w732:T5)
        }
        frame 1030 {
          w746 = 1.0 ("factor 1")
          # "Vdc"
          n483 = call "U8arrayToMeasurement.vi"("factor 2"=w746, "factor 1"=w746, "payload"=w745) -> ("Meas 2"=w743:dbl, "Meas 1"=w744:dbl)
          n484 = Add(x=w744, y=w743) -> (x+y=w739:dbl)
          n485 = Bundle By Name(cluster=w740, "Vdc4"=w739) -> (w741:T5)
        }
      }
      n486 = local write "measurements"(w571) -> ()
      n487 = local write "conv"(w573) -> ()
      "CAN IN" <- w575
    }
    n488 = local read "main stop"() -> (w567:bool)
    n489 = node-c288() -> ()  [unwired: 1 in, 1 out]
  }
  n490 = call <instrlib>:"niSync Close.vi"("error in (no error)"=w15, "instrument handle"=w16) -> ("error out"=→"Error out":errorcluster)  [unwired: 9 in]
  n491 = UDP Close(connection ID=w3, 8:w8) -> ()  [unwired: 2 out]
  n492 = while {
    stop <- w749 stop-if-true
    n493 = flat-sequence {
      tunnel: [w752] -> w750
      tunnel: w750 -> [w759]
      frame #0 {
        n494 = local read "start following 1 pre"() -> (w751:bool)
        n495 = call <userlib>:"Boolean Trigger__ogtk.vi"("Boolean Input"=w751) -> ("Rising Edge"=w753:bool)  [unwired: 1 in, 1 out]
        n496 = case shown="False" w753 {
          tunnel: w751 -> [w755 w756]
          tunnel: [w755 w756] -> w752
          frame False {
            n497 = Wait (ms)(milliseconds to wait=u32 50) -> ()  [unwired: 1 out]
          }
          frame True {
            n498 = Get Date/Time In Seconds() -> (seconds since 1Jan1904=→"time_afe":timestamp)
            n499 = Wait (ms)(milliseconds to wait=u32 550) -> ()  [unwired: 1 out]
          }
        }
      }
      frame #1 {
        n500 = local write "Start following 1"(w759) -> ()
      }
    }
    n501 = local read "main stop"() -> (w749:bool)
  }
  n502 = node-c288(w34) -> ()  [unwired: 1 out]
  n503 = node-c288(w29) -> ()  [unwired: 1 out]
  n504 = call <vilib>:"XNET Stop.vi"("session in"=w39) -> ()  [unwired: 13 in, 2 out]
  n505 = UDP Close(connection ID=w9, 8:w2) -> ()  [unwired: 2 out]
  n506 = local write "CAN with Conv"(w37) -> ()
  n507 = call <vilib>:"XNET Stop.vi"("session in"=w40) -> ()  [unwired: 13 in, 2 out]
  "Measurements" <- w26
  "CAN with Conv" <- w26
  "logging" <- w26
  "Ready 1" <- w26
  "OFF 1" <- w26
  "Ready 2" <- w26
  "ON 2" <- w26
  "OFF 2" <- w26
  "Ready 4" <- w26
  "ON 4" <- w26
  "OFF 4" <- w26
  "ON 3" <- w26
  "Ready 3" <- w26
  "OFF 3" <- w26
  "Fault 1" <- w26
  "Error 1" <- w26
  "Fault 2" <- w26
  "Error 2" <- w26
  "Fault 3" <- w26
  "Error 3" <- w26
  "Fault 4" <- w26
  "Error 4" <- w26
  "Forming 2" <- w23
  "Forming 1" <- w23
